vi "Group Analyser.vi"() -> ()   [LabVIEW 2016]
uses:
  Group Analyser state.ctl
  comm/comm.lvlib
  comm/impulse/impulse functions.lvlib
panel:
  in  "Fixed Time":bool
  in  "Fixed Time":bool
  in  "Active Plot":u16(ring) items=["BOTTOM PLOT", "TOP PLOT"]
  in  "Old Channels / Subject":T1(array[cluster])=[[{"Start"=0, "End"=1000000, "Offset"=0.0, "Deleted"=FALSE}]] {"Offset" format="%.2f"}
  in  "Channels / Subject":T1(array[cluster])=[[{"Start"=0, "End"=1000000, "Offset"=0.0, "Deleted"=FALSE}]] {"Offset" format="%.2f"}
  in  "Vertical Align to Zero":bool
  in  "Fixed Amplitude":bool
  out "Impulse Trace":cluster{dbl, dbl, dbl[][]}(graph)
  in  "Selected Files Text":string[](array[string])
  in  "Data Input":T2(array[cluster]) {"Data Channels" format="%.2f"}
  in  "Listbox":i32[](listbox)
  in  "Group Analyser":bool
  in  "Export Data":bool
  in  "Aligning Channel":u16(ring)=6 items=["Rx Position-in-Space", "Ry Position-in-Space", "Rz Position-in-Space", "Rx Velocity-in-Space", "Ry Velocity-in-Space", "Rz Velocity-in-Space", "Rl Velocity-in-Space", "Rr Velocity-in-Space", "Rx Acceleration-in-Space", "Ry Acceleration-in-Space", "Rz Acceleration-in-Space", "Rl Acceleration-in-Space", "Rr Acceleration-in-Space", "Chair Position", "Chair Velocity", " "]
  in  "Trigger Channel":u16(ring) items=["Rx Position-in-Space", "Ry Position-in-Space", "Rz Position-in-Space", "Rx Velocity-in-Space", "Ry Velocity-in-Space", "Rz Velocity-in-Space", "Rl Velocity-in-Space", "Rr Velocity-in-Space", "Rx Acceleration-in-Space", "Ry Acceleration-in-Space", "Rz Acceleration-in-Space", "Rl Acceleration-in-Space", "Rr Acceleration-in-Space", "Chair Position", "Chair Velocity", " "]
  in  "Plot Selection 2":T3(array[cluster])=[{"Color Box"=4652800, "Boolean"=TRUE, "List 2"=7, "Boolean 2"=FALSE}, {"Color Box"=16733696, "Boolean"=TRUE, "List 2"=15, "Boolean 2"=TRUE}, {"Color Box"=393436, "Boolean"=TRUE, "List 2"=23, "Boolean 2"=TRUE}] {"List 2" items=["Rx Position-in-Space", "Ry Position-in-Space", "Rz Position-in-Space", "Rx Velocity-in-Space", "Ry Velocity-in-Space", "Rz Velocity-in-Space", "Rl Velocity-in-Space", "Rr Velocity-in-Space", "Rx Acceleration-in-Space", "Ry Acceleration-in-Space", "Rz Acceleration-in-Space", "Rl Acceleration-in-Space", "Rr Acceleration-in-Space", "Chair Position", "Chair Velocity", " "]}
  in  "Select An  Other Trigger":bool
  in  "Group \nAnalyser":bool
  out "Processing":bool
  in  "View Impulse Parameters":bool
  in  "Filter Data":bool
  in  "View Filter Parameters":bool
  in  "Read Files":bool
  in  "Impulse Analyser":bool
  in  "Filter characteristics":T4={"Filter type"=enum."Lowpass", "Order"=50, "Higher pass freq"=40.0, "Lower pass freq"=40.0} {"Lower pass freq" format="%.2f"; "Higher pass freq" format="%.2f"}
  in  "Mean and STD":bool
  in  "Fixed Amplitude":bool
  in  "Cut After":bool
  in  "Cut Before":bool
  in  "Undo Last":bool
  in  "Delete Impulse":bool
  out "Impulse Trace":cluster{dbl, dbl, dbl[][]}(graph)
  in  "Vertical Align":bool
  in  "Horizontal Align":bool
  in  "Generate New Impulse Plot":bool
  in  "Select Files":bool
  in  "Plot Selection":T5(array[cluster])=[{"Color Box"=61223, "Boolean"=TRUE, "List 1"=5, "Boolean 2"=FALSE}, {"Color Box"=16722176, "Boolean"=TRUE, "List 1"=6, "Boolean 2"=FALSE}, {"Color Box"=6143, "Boolean"=TRUE, "List 1"=7, "Boolean 2"=FALSE}] {"List 1" items=["Rx Position-in-Space", "Ry Position-in-Space", "Rz Position-in-Space", "Rx Velocity-in-Space", "Ry Velocity-in-Space", "Rz Velocity-in-Space", "Rl Velocity-in-Space", "Rr Velocity-in-Space", "Rx Acceleration-in-Space", "Ry Acceleration-in-Space", "Rz Acceleration-in-Space", "Rl Acceleration-in-Space", "Rr Acceleration-in-Space", "Chair Position", "Chair Velocity", " "]}
  in  "Quit":bool
  in  "Stop":bool
  # "Copyright Americo A. Migliaccio (c) 2002 All Rights Reserved by Author"
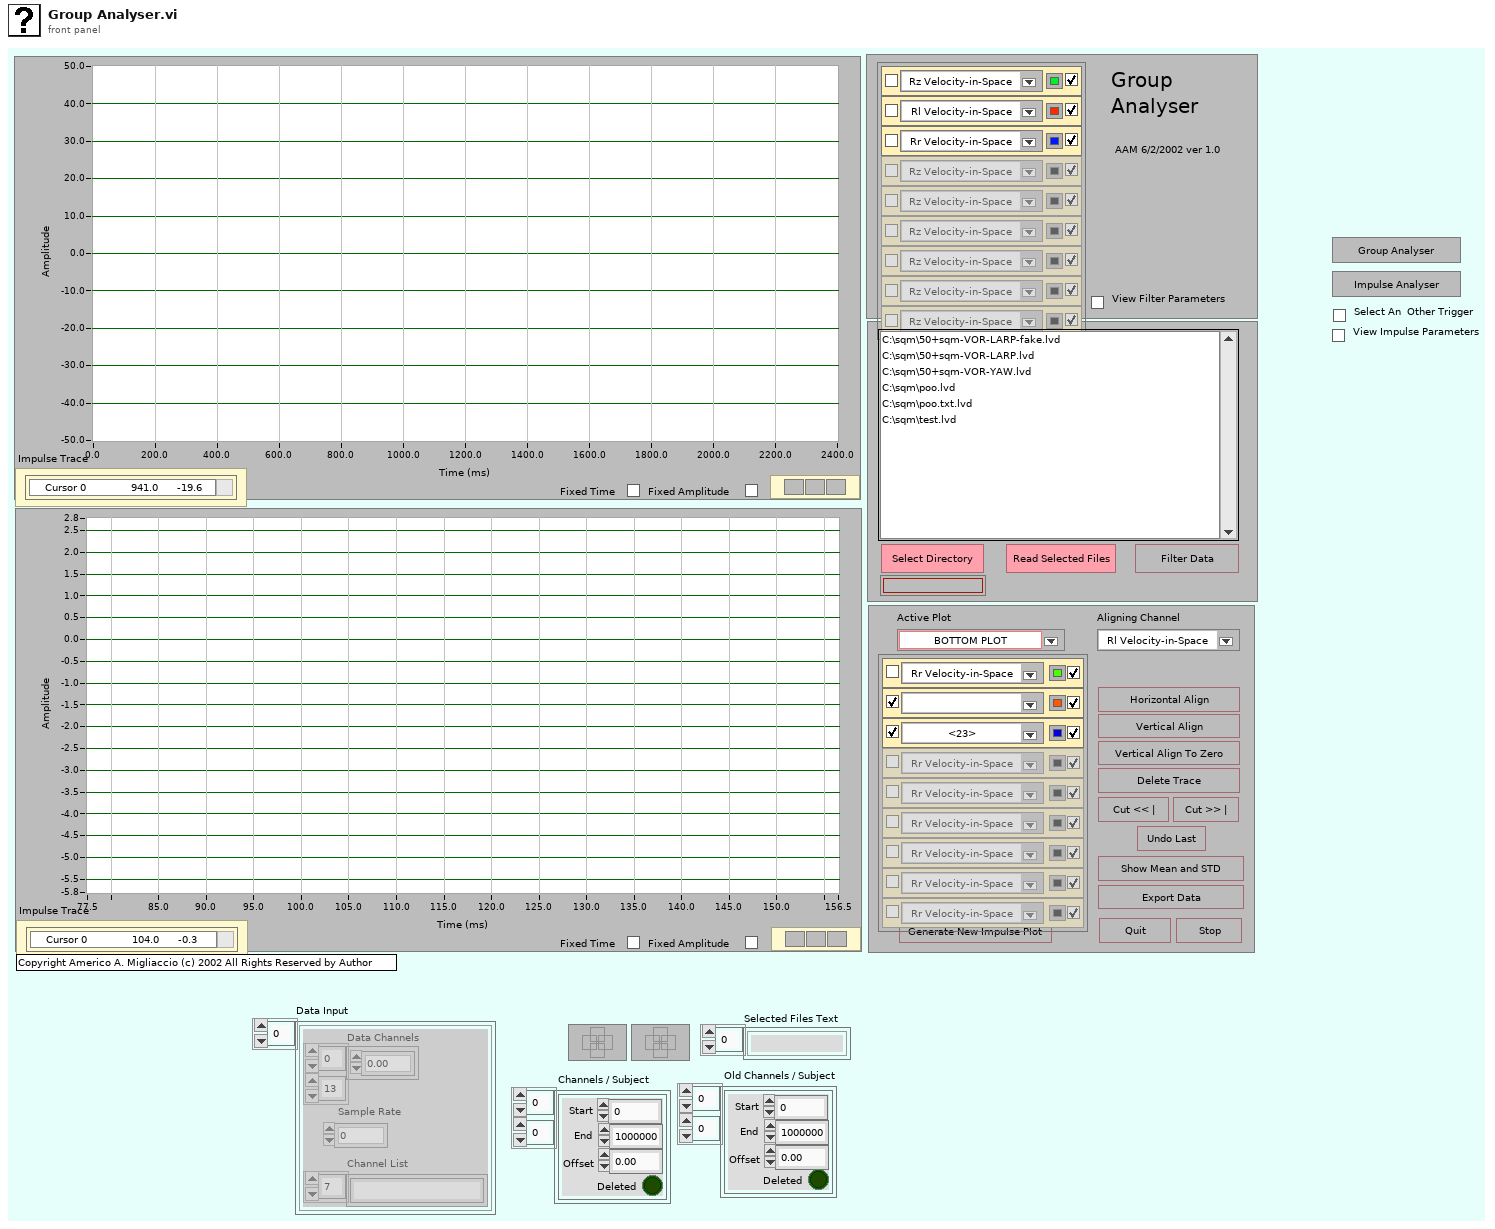
[diagram p1: front panel]
types:
  T1 = cluster{"Start":i32, "End":i32, "Offset":dbl, "Deleted":bool}[][]
  T2 = cluster{"Data Channels":dbl[][], "Sample Rate":i32, "Channel List":string[]}[]
  T3 = cluster{"Color Box":u32, "Boolean":bool, "List 2":u16, "Boolean 2":bool}[]
  T4 = cluster{"Filter type":enum32{"Lowpass", "Highpass", "Bandpass", "Bandstop"}, "Order":i32, "Higher pass freq":dbl, "Lower pass freq":dbl}
  T5 = cluster{"Color Box":u32, "Boolean":bool, "List 1":u16, "Boolean 2":bool}[]
  T6 = typedef "Group Analyser state.ctl" = enum16{"Panel Monitoring", "Read Files", "Select Files", "Generate New Impulse Plot", "Impulse Analyser", "Horizontal Align", "Vertical Align", "Vertical Align to Zero", "Delete Trace", "Cut Before", "Cut After", "Filter Data", "Undo Last", "Mean and STD", "Generate Report", "Export Data", "Initialize", "Stop", "Quit"}
  T7 = cluster{"Start":i32, "End":i32, "Offset":i32, "Deleted":bool}
  T8 = enum16{"open", "open or create", "create or replace", "create", "open (read only)"}
  T9 = cluster{"Data Input":cluster{"Data Channels":dbl[][], "Sample Rate":i32, "Channel List":string[]}[], "Selected Files Text":string[], " Channels / Subject":cluster{"Start":i32, "End":i32, "Offset":dbl, "Deleted":bool}[][], " Old Channels / Subject":cluster{"Start":i32, "End":i32, "Offset":dbl, "Deleted":bool}[][]}
  T10 = cluster{"Stop ":bool, "Quit":bool, "Read Files":bool, "Impulse Analyser":bool, "Select Files":bool, "View Filter Parameters":bool, "Filter Data":bool, "Generate New Impulse Plot":bool, "Vertical Align to Zero":bool, "Horizontal Align":bool, "Vertical Align":bool, "Delete Impulse":bool, "Undo Last":bool, "Cut Before":bool, "Cut After":bool, "Mean and STD":bool, "Select An  Other Trigger":bool, "Export Data":bool}
  T11 = enum32{"existing file", "new file", "new or existing file", "existing dir", "new dir", "new or existing dir", "existing file (use LLBs)", "new file (use LLBs)", "new or existing file (use LLBs)", "new or existing file or directory (use LLBs)"}
  T12 = cluster{"Data Channels":dbl[][], "Sample Rate":i32, "Channel List":string[]}
  T13 = cluster{"Start":i32, "End":i32, "Offset":i32, "Deleted":bool}[][]
  T14 = enum32{"Lowpass", "Highpass", "Bandpass", "Bandstop"}
  T15 = cluster{"Start":i32, "End":i32, "Offset":dbl, "Deleted":bool}
  T16 = cluster{"Color Box":u32, "Boolean":bool, "List 2":u16, "Boolean 2":bool}
  T17 = cluster{"Color Box":u32, "Boolean":bool, "List 1":u16, "Boolean 2":bool}
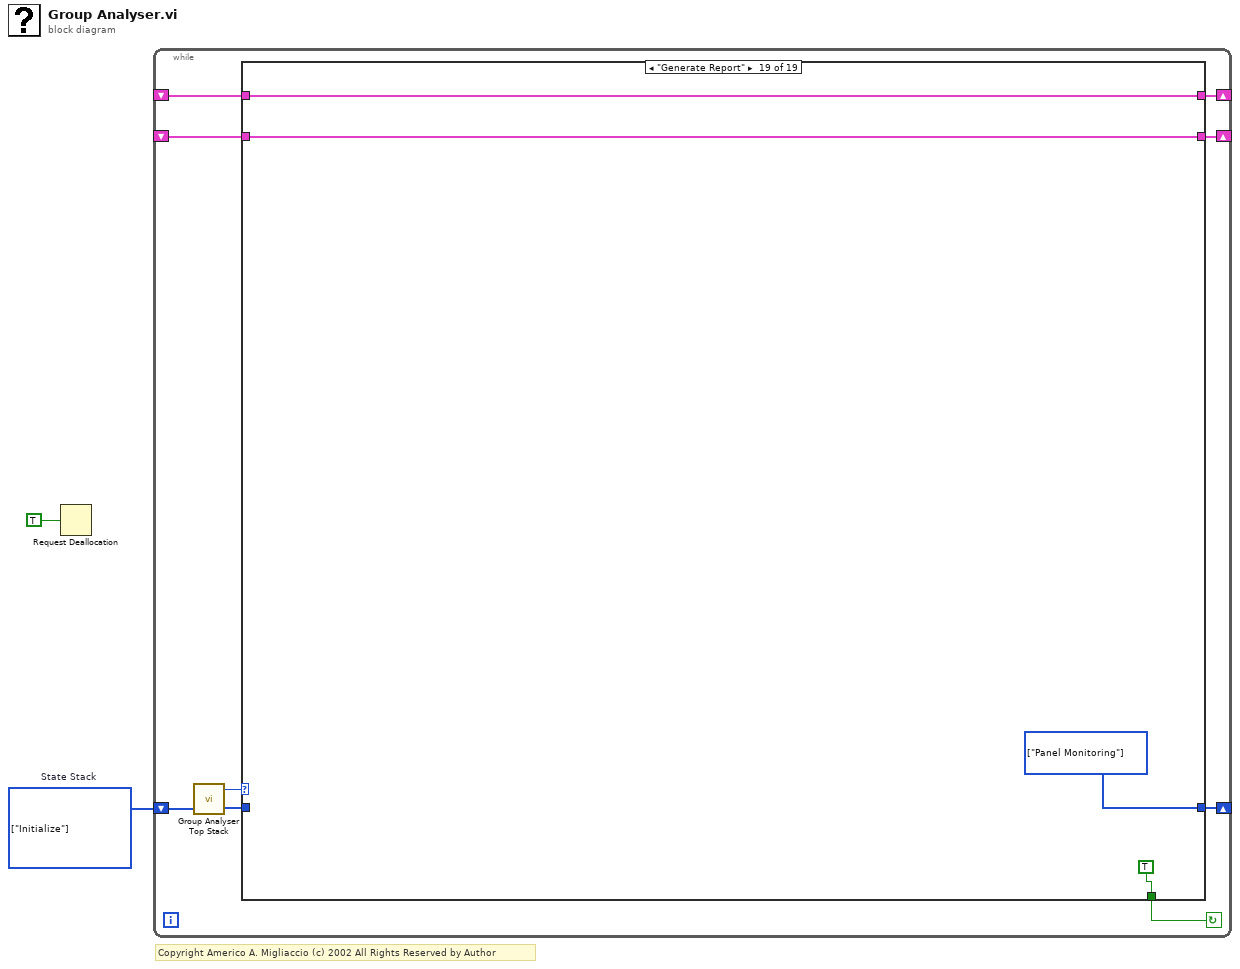
[diagram p0: block diagram]
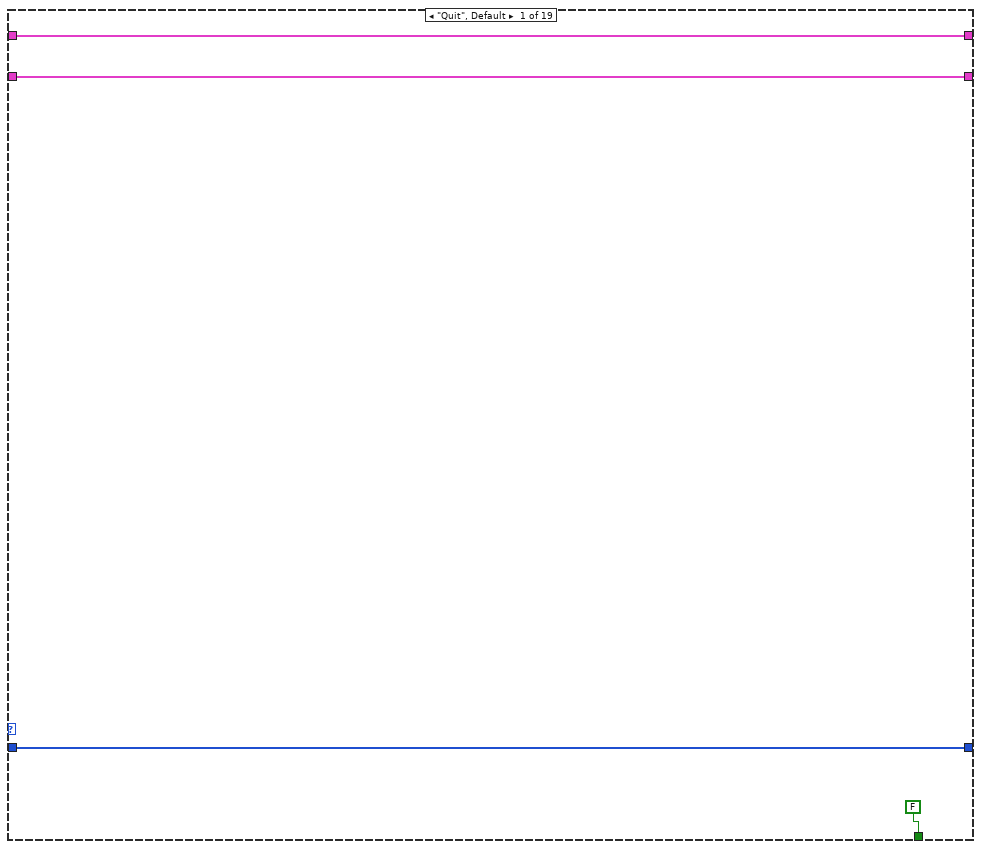
[diagram p2: hidden frame]
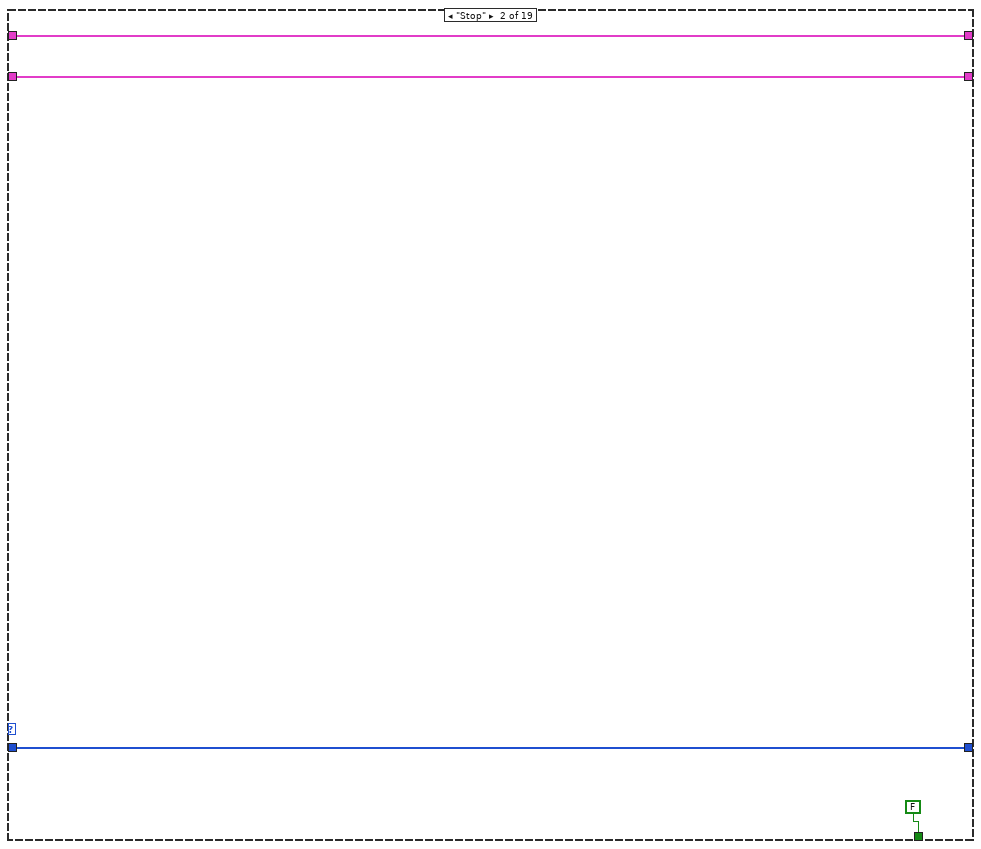
[diagram p3: hidden frame]
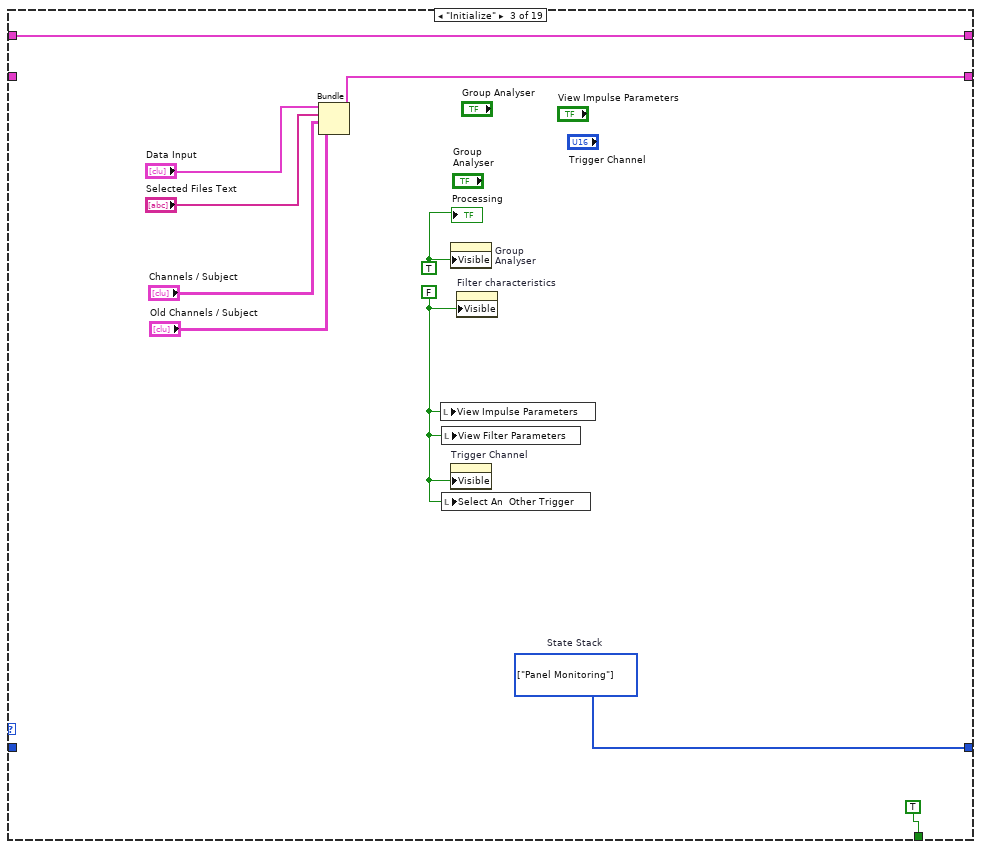
[diagram p4: hidden frame]
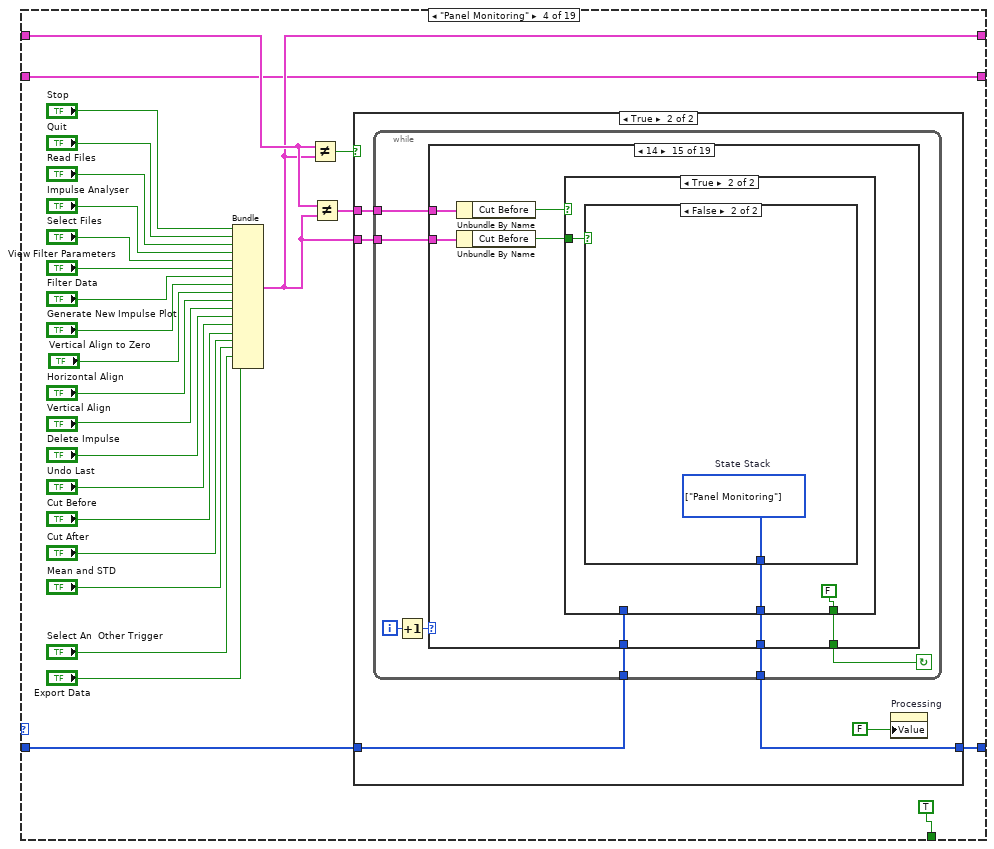
[diagram p5: hidden frame]
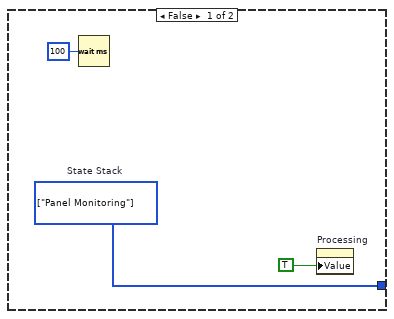
[diagram p6: hidden frame]
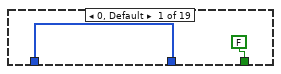
[diagram p7: hidden frame]
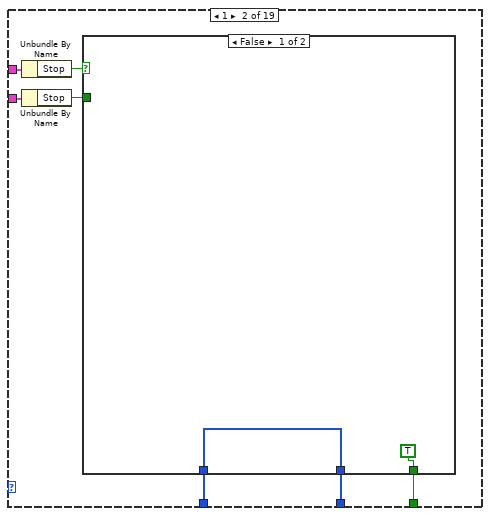
[diagram p8: hidden frame]
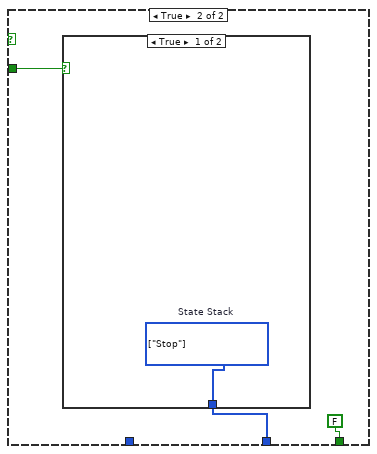
[diagram p9: hidden frame]
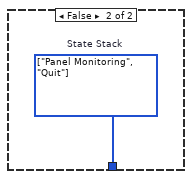
[diagram p10: hidden frame]
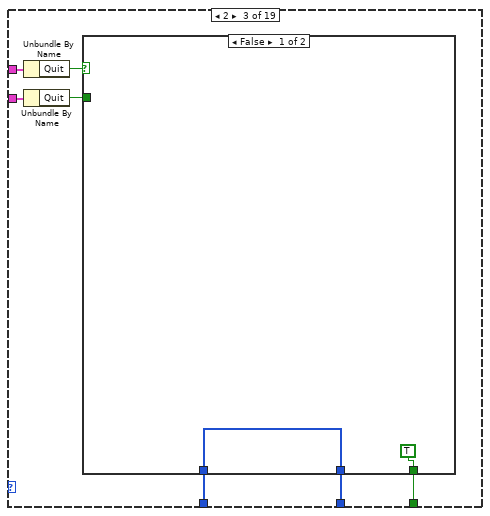
[diagram p11: hidden frame]
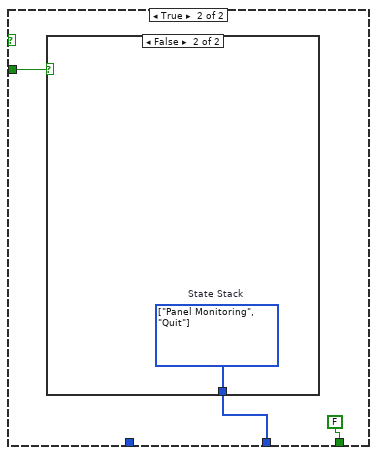
[diagram p12: hidden frame]
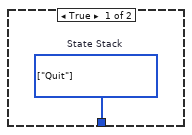
[diagram p13: hidden frame]
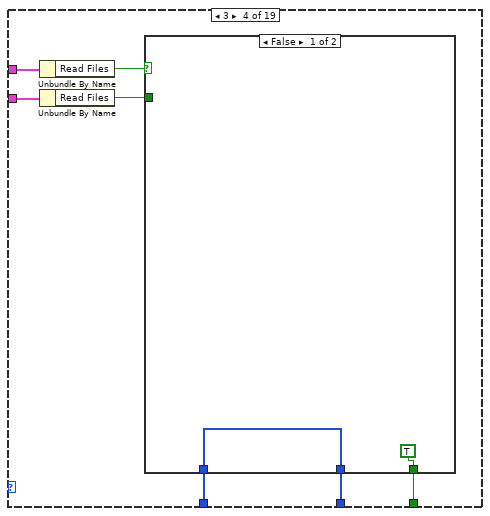
[diagram p14: hidden frame]
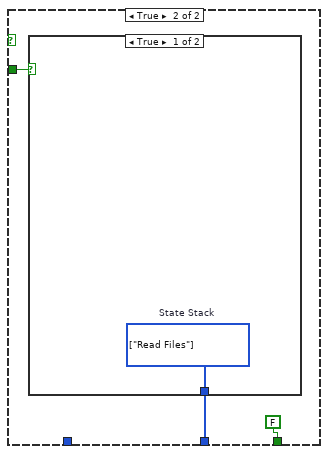
[diagram p15: hidden frame]
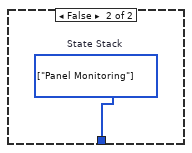
[diagram p16: hidden frame]
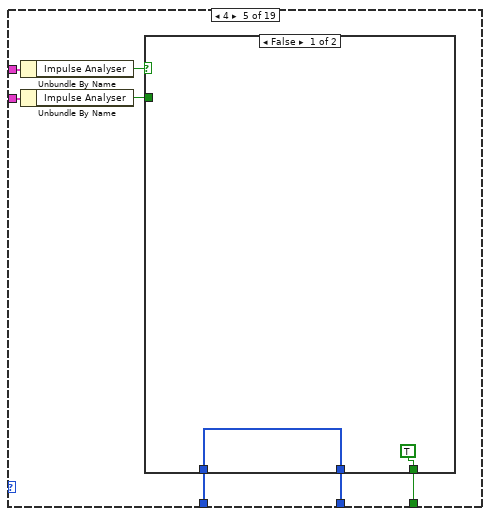
[diagram p17: hidden frame]
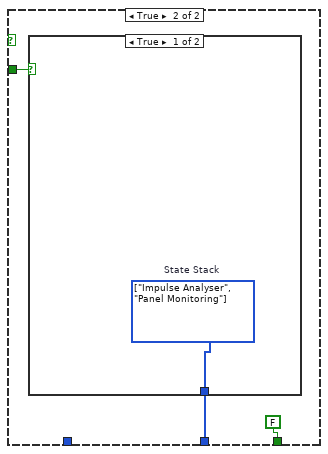
[diagram p18: hidden frame]
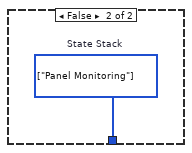
[diagram p19: hidden frame]
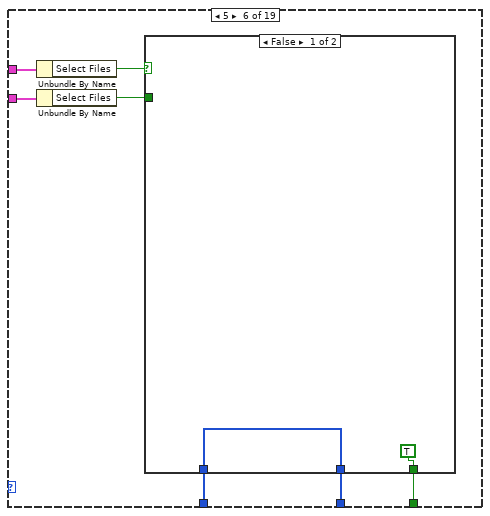
[diagram p20: hidden frame]
diagram:
  w2 = T6[] [enum."Initialize"] items=["Panel Monitoring", "Read Files", "Select Files", "Generate New Impulse Plot", "Impulse Analyser", "Horizontal Align", "Vertical Align", "Vertical Align to Zero", "Delete Trace", "Cut Before", "Cut After", "Filter Data", "Undo Last", "Mean and STD", "Generate Report", "Export Data", "Initialize", "Stop", "Quit"]  # State Stack
  # "Copyright Americo A. Migliaccio (c) 2002 All Rights Reserved by Author"
  n1 = Request Deallocation(TRUE ("flag")) -> ()
  n2 = while {
    shift-left: _ -> [w4]
    shift-right: [w5] -> _
    shift-left: _ -> [w7]
    shift-right: [w8] -> _
    shift-left: w2 -> [w11]
    shift-right: [w9] -> _
    stop <- w6 continue-if-true
    n3 = call "Group Analyser Top Stack.vi"("State Stack (in)"=w11) -> ("State Stack (out)"=w10:T6[], "State"=w3:T6)  [unwired: 1 in]
    n4 = case shown="\"Generate Report\"" w3 {
      tunnel: w10 -> [w15 w19 _ w50 _ _ w375 _ w490 w507 w522 w538 w570 w592 w610 _ w695 _ _]
      tunnel: [w15 w19 w28 w49 w335 w357 w375 w403 w490 w507 w522 w538 w570 w592 w610 w636 w695 w742 w753] -> w9
      tunnel: [w13 w17 w27 w46 w336 w358 w382 w404 w491 w508 w523 w540 w571 w595 w611 w637 w696 w743 w754] -> w8
      tunnel: w7 -> [w13 w17 w27 w52 w336 w358 w382 w404 w491 w508 w523 w540 w571 w595 w611 w637 w696 w743 w754]
      tunnel: [FALSE FALSE TRUE TRUE TRUE TRUE TRUE TRUE TRUE TRUE TRUE TRUE TRUE TRUE TRUE TRUE TRUE TRUE TRUE] -> w6
      tunnel: [w12 w16 w24 w33 w326 w350 w372 w398 w488 w503 w519 w539 w562 w593 w608 w631 w694 w741 w752] -> w5
      tunnel: w4 -> [w12 w16 _ w33 w328 w356 w373 w398 w489 w504 w520 w537 w563 w594 w609 w631 w694 w741 w752]
      frame "Quit", Default {
      }
      frame "Stop" {
      }
      frame "Initialize" {
        w28 = T6[] [enum."Panel Monitoring"] items=["Panel Monitoring", "Read Files", "Select Files", "Generate New Impulse Plot", "Impulse Analyser", "Horizontal Align", "Vertical Align", "Vertical Align to Zero", "Delete Trace", "Cut Before", "Cut After", "Filter Data", "Undo Last", "Mean and STD", "Generate Report", "Export Data", "Initialize", "Stop", "Quit"]  # State Stack
        w26 = TRUE ("Visible")
        w25 = FALSE
        n5 = Bundle("Data Input"="Data Input", "Selected Files Text"="Selected Files Text", "Channels / Subject"="Channels / Subject", "Old Channels / Subject"="Old Channels / Subject") -> (w24:T9)  [unwired: 1 in]
        n6 = local write "View Impulse Parameters"(w25) -> ()
        n7 = local write "View Filter Parameters"(w25) -> ()
        n8 = local write "Select An  Other Trigger"(w25) -> ()
        n9 = property on="Group \nAnalyser" class="Bool"("Visible"=w26) -> ()  [unwired: 2 in, 2 out]
        n10 = property on="Trigger Channel" class="Ring (strict)"("Visible"=w25) -> ()  [unwired: 2 in, 2 out]
        n11 = property on="Filter characteristics" class="Clust (strict)"("Visible"=w25) -> ()  [unwired: 2 in, 2 out]
        "Processing" <- w26
      }
      frame "Panel Monitoring" {
        n12 = Bundle("Stop"="Stop", "Quit"="Quit", "Read Files"="Read Files", "Impulse Analyser"="Impulse Analyser", "Select Files"="Select Files", "View Filter Parameters"="View Filter Parameters", "Filter Data"="Filter Data", "Generate New Impulse Plot"="Generate New Impulse Plot", "Vertical Align to Zero"="Vertical Align to Zero", "Horizontal Align"="Horizontal Align", "Vertical Align"="Vertical Align", "Delete Impulse"="Delete Impulse", "Undo Last"="Undo Last", "Cut Before"="Cut Before", "Cut After"="Cut After", "Mean and STD"="Mean and STD", "Select An  Other Trigger"="Select An  Other Trigger", "Export Data"="Export Data") -> (w46:T10)  [unwired: 1 in]
        n13 = Not Equal?(x=w52, y=w46) -> (x != y?=w53:bool)
        n14 = Not Equal?(x=w52, y=w46) -> (x != y?=w51:T10)
        n15 = case shown="True" w53 {
          tunnel: w51 -> [_ w63]
          tunnel: w50 -> [_ w61]
          tunnel: [w58 w62] -> w49
          tunnel: w46 -> [_ w60]
          frame False {
            w58 = T6[] [enum."Panel Monitoring"] items=["Panel Monitoring", "Read Files", "Select Files", "Generate New Impulse Plot", "Impulse Analyser", "Horizontal Align", "Vertical Align", "Vertical Align to Zero", "Delete Trace", "Cut Before", "Cut After", "Filter Data", "Undo Last", "Mean and STD", "Generate Report", "Export Data", "Initialize", "Stop", "Quit"]  # State Stack
            n16 = Wait (ms)(milliseconds to wait=u32 100) -> ()  [unwired: 1 out]
            n17 = property on="Processing" class="Bool (strict)"("Value"=TRUE) -> ()  [unwired: 2 in, 2 out]
          }
          frame True {
            n18 = while {
              tunnel: w60 -> [w64]
              tunnel: w61 -> [w67]
              tunnel: [w68] -> w62
              tunnel: w63 -> [w70]
              i -> [w69]
              stop <- w66 continue-if-true
              n19 = Increment(x=w69) -> (x+1=w65:i32)
              n20 = case shown="14" w65 {
                tunnel: w70 -> [_ w79 w93 w107 w121 w135 w149 w162 w176 w190 w204 w218 w232 w246 w260 w274 w288 w303 w317]
                tunnel: [w72 w77 w91 w105 w119 w133 w147 w160 w174 w188 w202 w216 w230 w244 w258 w272 w286 w301 w315] -> w68
                tunnel: w67 -> [w72 w76 w90 w104 w118 w132 w146 w159 w173 w187 w201 w215 w229 w243 w257 w271 w285 w300 w314]
                tunnel: [FALSE w75 w89 w103 w117 w131 w145 w158 w172 w186 w200 w214 w228 w242 w256 w270 w284 w299 w313] -> w66
                tunnel: w64 -> [_ w74 w88 w102 w116 w130 w144 w157 w171 w185 w199 w213 w227 w241 w255 w269 w283 w298 w312]
                frame 0, Default {
                }
                frame 1 {
                  n21 = Unbundle By Name(w79) -> ("Stop"=w78:bool)
                  n22 = Unbundle By Name(w74) -> ("Stop"=w73:bool)
                  n23 = case shown="False" w78 {
                    tunnel: [w81 w84] -> w77
                    tunnel: w76 -> [w81 _]
                    tunnel: [TRUE FALSE] -> w75
                    tunnel: w73 -> [_ w82]
                    frame False {
                    }
                    frame True {
                      n24 = case shown="True" w82 {
                        tunnel: [w85 w86] -> w84
                        frame True {
                          w85 = T6[] [enum."Stop"] items=["Panel Monitoring", "Read Files", "Select Files", "Generate New Impulse Plot", "Impulse Analyser", "Horizontal Align", "Vertical Align", "Vertical Align to Zero", "Delete Trace", "Cut Before", "Cut After", "Filter Data", "Undo Last", "Mean and STD", "Generate Report", "Export Data", "Initialize", "Stop", "Quit"]  # State Stack
                        }
                        frame False {
                          w86 = T6[] [enum."Panel Monitoring", enum."Quit"] items=["Panel Monitoring", "Read Files", "Select Files", "Generate New Impulse Plot", "Impulse Analyser", "Horizontal Align", "Vertical Align", "Vertical Align to Zero", "Delete Trace", "Cut Before", "Cut After", "Filter Data", "Undo Last", "Mean and STD", "Generate Report", "Export Data", "Initialize", "Stop", "Quit"]  # State Stack
                        }
                      }
                    }
                  }
                }
                frame 2 {
                  n25 = Unbundle By Name(w93) -> ("Quit"=w92:bool)
                  n26 = Unbundle By Name(w88) -> ("Quit"=w87:bool)
                  n27 = case shown="False" w92 {
                    tunnel: [w95 w98] -> w91
                    tunnel: w90 -> [w95 _]
                    tunnel: [TRUE FALSE] -> w89
                    tunnel: w87 -> [_ w96]
                    frame False {
                    }
                    frame True {
                      n28 = case shown="False" w96 {
                        tunnel: [w99 w100] -> w98
                        frame True {
                          w99 = T6[] [enum."Quit"] items=["Panel Monitoring", "Read Files", "Select Files", "Generate New Impulse Plot", "Impulse Analyser", "Horizontal Align", "Vertical Align", "Vertical Align to Zero", "Delete Trace", "Cut Before", "Cut After", "Filter Data", "Undo Last", "Mean and STD", "Generate Report", "Export Data", "Initialize", "Stop", "Quit"]  # State Stack
                        }
                        frame False {
                          w100 = T6[] [enum."Panel Monitoring", enum."Quit"] items=["Panel Monitoring", "Read Files", "Select Files", "Generate New Impulse Plot", "Impulse Analyser", "Horizontal Align", "Vertical Align", "Vertical Align to Zero", "Delete Trace", "Cut Before", "Cut After", "Filter Data", "Undo Last", "Mean and STD", "Generate Report", "Export Data", "Initialize", "Stop", "Quit"]  # State Stack
                        }
                      }
                    }
                  }
                }
                frame 3 {
                  n29 = Unbundle By Name(w107) -> ("Read Files"=w106:bool)
                  n30 = Unbundle By Name(w102) -> ("Read Files"=w101:bool)
                  n31 = case shown="False" w106 {
                    tunnel: [w109 w112] -> w105
                    tunnel: w104 -> [w109 _]
                    tunnel: [TRUE FALSE] -> w103
                    tunnel: w101 -> [_ w110]
                    frame False {
                    }
                    frame True {
                      n32 = case shown="True" w110 {
                        tunnel: [w113 w114] -> w112
                        frame True {
                          w113 = T6[] [enum."Read Files"] items=["Panel Monitoring", "Read Files", "Select Files", "Generate New Impulse Plot", "Impulse Analyser", "Horizontal Align", "Vertical Align", "Vertical Align to Zero", "Delete Trace", "Cut Before", "Cut After", "Filter Data", "Undo Last", "Mean and STD", "Generate Report", "Export Data", "Initialize", "Stop", "Quit"]  # State Stack
                        }
                        frame False {
                          w114 = T6[] [enum."Panel Monitoring"] items=["Panel Monitoring", "Read Files", "Select Files", "Generate New Impulse Plot", "Impulse Analyser", "Horizontal Align", "Vertical Align", "Vertical Align to Zero", "Delete Trace", "Cut Before", "Cut After", "Filter Data", "Undo Last", "Mean and STD", "Generate Report", "Export Data", "Initialize", "Stop", "Quit"]  # State Stack
                        }
                      }
                    }
                  }
                }
                frame 4 {
                  n33 = Unbundle By Name(w121) -> ("Impulse Analyser"=w120:bool)
                  n34 = Unbundle By Name(w116) -> ("Impulse Analyser"=w115:bool)
                  n35 = case shown="False" w120 {
                    tunnel: [w123 w126] -> w119
                    tunnel: w118 -> [w123 _]
                    tunnel: [TRUE FALSE] -> w117
                    tunnel: w115 -> [_ w124]
                    frame False {
                    }
                    frame True {
                      n36 = case shown="True" w124 {
                        tunnel: [w127 w128] -> w126
                        frame True {
                          w127 = T6[] [enum."Impulse Analyser", enum."Panel Monitoring"] items=["Panel Monitoring", "Read Files", "Select Files", "Generate New Impulse Plot", "Impulse Analyser", "Horizontal Align", "Vertical Align", "Vertical Align to Zero", "Delete Trace", "Cut Before", "Cut After", "Filter Data", "Undo Last", "Mean and STD", "Generate Report", "Export Data", "Initialize", "Stop", "Quit"]  # State Stack
                        }
                        frame False {
                          w128 = T6[] [enum."Panel Monitoring"] items=["Panel Monitoring", "Read Files", "Select Files", "Generate New Impulse Plot", "Impulse Analyser", "Horizontal Align", "Vertical Align", "Vertical Align to Zero", "Delete Trace", "Cut Before", "Cut After", "Filter Data", "Undo Last", "Mean and STD", "Generate Report", "Export Data", "Initialize", "Stop", "Quit"]  # State Stack
                        }
                      }
                    }
                  }
                }
                frame 5 {
                  n37 = Unbundle By Name(w135) -> ("Select Files"=w134:bool)
                  n38 = Unbundle By Name(w130) -> ("Select Files"=w129:bool)
                  n39 = case shown="False" w134 {
                    tunnel: [w137 w140] -> w133
                    tunnel: w132 -> [w137 _]
                    tunnel: [TRUE FALSE] -> w131
                    tunnel: w129 -> [_ w138]
                    frame False {
                    }
                    frame True {
                      n40 = case shown="True" w138 {
                        tunnel: [w141 w142] -> w140
                        frame True {
                          w141 = T6[] [enum."Select Files"] items=["Panel Monitoring", "Read Files", "Select Files", "Generate New Impulse Plot", "Impulse Analyser", "Horizontal Align", "Vertical Align", "Vertical Align to Zero", "Delete Trace", "Cut Before", "Cut After", "Filter Data", "Undo Last", "Mean and STD", "Generate Report", "Export Data", "Initialize", "Stop", "Quit"]  # State Stack
                        }
                        frame False {
                          w142 = T6[] [enum."Panel Monitoring"] items=["Panel Monitoring", "Read Files", "Select Files", "Generate New Impulse Plot", "Impulse Analyser", "Horizontal Align", "Vertical Align", "Vertical Align to Zero", "Delete Trace", "Cut Before", "Cut After", "Filter Data", "Undo Last", "Mean and STD", "Generate Report", "Export Data", "Initialize", "Stop", "Quit"]  # State Stack
                        }
                      }
                    }
                  }
                }
                frame 6 {
                  n41 = Unbundle By Name(w149) -> ("View Filter Parameters"=w148:bool)
                  n42 = Unbundle By Name(w144) -> ("View Filter Parameters"=w143:bool)
                  n43 = case shown="True" w148 {
                    tunnel: [w151 w154] -> w147
                    tunnel: w146 -> [w151 _]
                    tunnel: [TRUE FALSE] -> w145
                    tunnel: w143 -> [_ w152]
                    frame False {
                    }
                    frame True {
                      w154 = T6[] [enum."Panel Monitoring"] items=["Panel Monitoring", "Read Files", "Select Files", "Generate New Impulse Plot", "Impulse Analyser", "Horizontal Align", "Vertical Align", "Vertical Align to Zero", "Delete Trace", "Cut Before", "Cut After", "Filter Data", "Undo Last", "Mean and STD", "Generate Report", "Export Data", "Initialize", "Stop", "Quit"]  # State Stack
                      n44 = Not(x=w152) -> (.not. x?=w153:bool)
                      n45 = property on="Filter characteristics" class="Clust (strict)"("Visible"=w152) -> ()  [unwired: 2 in, 2 out]
                      n46 = property on="Group \nAnalyser" class="Bool"("Visible"=w153) -> ()  [unwired: 2 in, 2 out]
                    }
                  }
                }
                frame 7 {
                  n47 = Unbundle By Name(w162) -> ("Filter Data"=w161:bool)
                  n48 = Unbundle By Name(w157) -> ("Filter Data"=w156:bool)
                  n49 = case shown="False" w161 {
                    tunnel: [w164 w167] -> w160
                    tunnel: w159 -> [w164 _]
                    tunnel: [TRUE FALSE] -> w158
                    tunnel: w156 -> [_ w165]
                    frame False {
                    }
                    frame True {
                      n50 = case shown="True" w165 {
                        tunnel: [w168 w169] -> w167
                        frame True {
                          w168 = T6[] [enum."Filter Data", enum."Select Files"] items=["Panel Monitoring", "Read Files", "Select Files", "Generate New Impulse Plot", "Impulse Analyser", "Horizontal Align", "Vertical Align", "Vertical Align to Zero", "Delete Trace", "Cut Before", "Cut After", "Filter Data", "Undo Last", "Mean and STD", "Generate Report", "Export Data", "Initialize", "Stop", "Quit"]  # State Stack
                        }
                        frame False {
                          w169 = T6[] [enum."Panel Monitoring"] items=["Panel Monitoring", "Read Files", "Select Files", "Generate New Impulse Plot", "Impulse Analyser", "Horizontal Align", "Vertical Align", "Vertical Align to Zero", "Delete Trace", "Cut Before", "Cut After", "Filter Data", "Undo Last", "Mean and STD", "Generate Report", "Export Data", "Initialize", "Stop", "Quit"]  # State Stack
                        }
                      }
                    }
                  }
                }
                frame 8 {
                  n51 = Unbundle By Name(w176) -> ("Generate New Impulse Plot"=w175:bool)
                  n52 = Unbundle By Name(w171) -> ("Generate New Impulse Plot"=w170:bool)
                  n53 = case shown="True" w175 {
                    tunnel: [w178 w181] -> w174
                    tunnel: w173 -> [w178 _]
                    tunnel: [TRUE FALSE] -> w172
                    tunnel: w170 -> [_ w179]
                    frame False {
                    }
                    frame True {
                      n54 = case shown="False" w179 {
                        tunnel: [w182 w183] -> w181
                        frame True {
                          w182 = T6[] [enum."Generate New Impulse Plot"] items=["Panel Monitoring", "Read Files", "Select Files", "Generate New Impulse Plot", "Impulse Analyser", "Horizontal Align", "Vertical Align", "Vertical Align to Zero", "Delete Trace", "Cut Before", "Cut After", "Filter Data", "Undo Last", "Mean and STD", "Generate Report", "Export Data", "Initialize", "Stop", "Quit"]  # State Stack
                        }
                        frame False {
                          w183 = T6[] [enum."Panel Monitoring"] items=["Panel Monitoring", "Read Files", "Select Files", "Generate New Impulse Plot", "Impulse Analyser", "Horizontal Align", "Vertical Align", "Vertical Align to Zero", "Delete Trace", "Cut Before", "Cut After", "Filter Data", "Undo Last", "Mean and STD", "Generate Report", "Export Data", "Initialize", "Stop", "Quit"]  # State Stack
                        }
                      }
                    }
                  }
                }
                frame 9 {
                  n55 = Unbundle By Name(w190) -> ("Vertical Align to Zero"=w189:bool)
                  n56 = Unbundle By Name(w185) -> ("Vertical Align to Zero"=w184:bool)
                  n57 = case shown="True" w189 {
                    tunnel: [w192 w194] -> w188
                    tunnel: w187 -> [w192 _]
                    tunnel: [TRUE FALSE] -> w186
                    tunnel: w184 -> [_ w193]
                    frame False {
                    }
                    frame True {
                      n58 = case shown="True" w193 {
                        tunnel: [w196 w197] -> w194
                        frame True {
                          w196 = T6[] [enum."Vertical Align to Zero", enum."Generate New Impulse Plot"] items=["Panel Monitoring", "Read Files", "Select Files", "Generate New Impulse Plot", "Impulse Analyser", "Horizontal Align", "Vertical Align", "Vertical Align to Zero", "Delete Trace", "Cut Before", "Cut After", "Filter Data", "Undo Last", "Mean and STD", "Generate Report", "Export Data", "Initialize", "Stop", "Quit"]  # State Stack
                        }
                        frame False {
                          w197 = T6[] [enum."Panel Monitoring"] items=["Panel Monitoring", "Read Files", "Select Files", "Generate New Impulse Plot", "Impulse Analyser", "Horizontal Align", "Vertical Align", "Vertical Align to Zero", "Delete Trace", "Cut Before", "Cut After", "Filter Data", "Undo Last", "Mean and STD", "Generate Report", "Export Data", "Initialize", "Stop", "Quit"]  # State Stack
                        }
                      }
                    }
                  }
                }
                frame 10 {
                  n59 = Unbundle By Name(w204) -> ("Horizontal Align"=w203:bool)
                  n60 = Unbundle By Name(w199) -> ("Horizontal Align"=w198:bool)
                  n61 = case shown="True" w203 {
                    tunnel: [w206 w209] -> w202
                    tunnel: w201 -> [w206 _]
                    tunnel: [TRUE FALSE] -> w200
                    tunnel: w198 -> [_ w207]
                    frame False {
                    }
                    frame True {
                      n62 = case shown="True" w207 {
                        tunnel: [w210 w211] -> w209
                        frame True {
                          w210 = T6[] [enum."Horizontal Align", enum."Generate New Impulse Plot"] items=["Panel Monitoring", "Read Files", "Select Files", "Generate New Impulse Plot", "Impulse Analyser", "Horizontal Align", "Vertical Align", "Vertical Align to Zero", "Delete Trace", "Cut Before", "Cut After", "Filter Data", "Undo Last", "Mean and STD", "Generate Report", "Export Data", "Initialize", "Stop", "Quit"]  # State Stack
                        }
                        frame False {
                          w211 = T6[] [enum."Panel Monitoring"] items=["Panel Monitoring", "Read Files", "Select Files", "Generate New Impulse Plot", "Impulse Analyser", "Horizontal Align", "Vertical Align", "Vertical Align to Zero", "Delete Trace", "Cut Before", "Cut After", "Filter Data", "Undo Last", "Mean and STD", "Generate Report", "Export Data", "Initialize", "Stop", "Quit"]  # State Stack
                        }
                      }
                    }
                  }
                }
                frame 11 {
                  n63 = Unbundle By Name(w218) -> ("Vertical Align"=w217:bool)
                  n64 = Unbundle By Name(w213) -> ("Vertical Align"=w212:bool)
                  n65 = case shown="True" w217 {
                    tunnel: [w220 w223] -> w216
                    tunnel: w215 -> [w220 _]
                    tunnel: [TRUE FALSE] -> w214
                    tunnel: w212 -> [_ w221]
                    frame False {
                    }
                    frame True {
                      n66 = case shown="True" w221 {
                        tunnel: [w224 w225] -> w223
                        frame True {
                          w224 = T6[] [enum."Vertical Align", enum."Generate New Impulse Plot"] items=["Panel Monitoring", "Read Files", "Select Files", "Generate New Impulse Plot", "Impulse Analyser", "Horizontal Align", "Vertical Align", "Vertical Align to Zero", "Delete Trace", "Cut Before", "Cut After", "Filter Data", "Undo Last", "Mean and STD", "Generate Report", "Export Data", "Initialize", "Stop", "Quit"]  # State Stack
                        }
                        frame False {
                          w225 = T6[] [enum."Panel Monitoring", enum."Quit"] items=["Panel Monitoring", "Read Files", "Select Files", "Generate New Impulse Plot", "Impulse Analyser", "Horizontal Align", "Vertical Align", "Vertical Align to Zero", "Delete Trace", "Cut Before", "Cut After", "Filter Data", "Undo Last", "Mean and STD", "Generate Report", "Export Data", "Initialize", "Stop", "Quit"]  # State Stack
                        }
                      }
                    }
                  }
                }
                frame 12 {
                  n67 = Unbundle By Name(w232) -> ("Delete Impulse"=w231:bool)
                  n68 = Unbundle By Name(w227) -> ("Delete Impulse"=w226:bool)
                  n69 = case shown="True" w231 {
                    tunnel: [w234 w237] -> w230
                    tunnel: w229 -> [w234 _]
                    tunnel: [TRUE FALSE] -> w228
                    tunnel: w226 -> [_ w235]
                    frame False {
                    }
                    frame True {
                      n70 = case shown="False" w235 {
                        tunnel: [w238 w239] -> w237
                        frame True {
                          w238 = T6[] [enum."Delete Trace", enum."Generate New Impulse Plot"] items=["Panel Monitoring", "Read Files", "Select Files", "Generate New Impulse Plot", "Impulse Analyser", "Horizontal Align", "Vertical Align", "Vertical Align to Zero", "Delete Trace", "Cut Before", "Cut After", "Filter Data", "Undo Last", "Mean and STD", "Generate Report", "Export Data", "Initialize", "Stop", "Quit"]  # State Stack
                        }
                        frame False {
                          w239 = T6[] [enum."Panel Monitoring"] items=["Panel Monitoring", "Read Files", "Select Files", "Generate New Impulse Plot", "Impulse Analyser", "Horizontal Align", "Vertical Align", "Vertical Align to Zero", "Delete Trace", "Cut Before", "Cut After", "Filter Data", "Undo Last", "Mean and STD", "Generate Report", "Export Data", "Initialize", "Stop", "Quit"]  # State Stack
                        }
                      }
                    }
                  }
                }
                frame 13 {
                  n71 = Unbundle By Name(w246) -> ("Undo Last"=w245:bool)
                  n72 = Unbundle By Name(w241) -> ("Undo Last"=w240:bool)
                  n73 = case shown="True" w245 {
                    tunnel: [w248 w251] -> w244
                    tunnel: w243 -> [w248 _]
                    tunnel: [TRUE FALSE] -> w242
                    tunnel: w240 -> [_ w249]
                    frame False {
                    }
                    frame True {
                      n74 = case shown="True" w249 {
                        tunnel: [w252 w253] -> w251
                        frame True {
                          w252 = T6[] [enum."Undo Last", enum."Generate New Impulse Plot"] items=["Panel Monitoring", "Read Files", "Select Files", "Generate New Impulse Plot", "Impulse Analyser", "Horizontal Align", "Vertical Align", "Vertical Align to Zero", "Delete Trace", "Cut Before", "Cut After", "Filter Data", "Undo Last", "Mean and STD", "Generate Report", "Export Data", "Initialize", "Stop", "Quit"]  # State Stack
                        }
                        frame False {
                          w253 = T6[] [enum."Panel Monitoring"] items=["Panel Monitoring", "Read Files", "Select Files", "Generate New Impulse Plot", "Impulse Analyser", "Horizontal Align", "Vertical Align", "Vertical Align to Zero", "Delete Trace", "Cut Before", "Cut After", "Filter Data", "Undo Last", "Mean and STD", "Generate Report", "Export Data", "Initialize", "Stop", "Quit"]  # State Stack
                        }
                      }
                    }
                  }
                }
                frame 14 {
                  n75 = Unbundle By Name(w260) -> ("Cut Before"=w259:bool)
                  n76 = Unbundle By Name(w255) -> ("Cut Before"=w254:bool)
                  n77 = case shown="True" w259 {
                    tunnel: [w262 w265] -> w258
                    tunnel: w257 -> [w262 _]
                    tunnel: [TRUE FALSE] -> w256
                    tunnel: w254 -> [_ w263]
                    frame False {
                    }
                    frame True {
                      n78 = case shown="False" w263 {
                        tunnel: [w266 w267] -> w265
                        frame True {
                          w266 = T6[] [enum."Cut Before", enum."Generate New Impulse Plot"] items=["Panel Monitoring", "Read Files", "Select Files", "Generate New Impulse Plot", "Impulse Analyser", "Horizontal Align", "Vertical Align", "Vertical Align to Zero", "Delete Trace", "Cut Before", "Cut After", "Filter Data", "Undo Last", "Mean and STD", "Generate Report", "Export Data", "Initialize", "Stop", "Quit"]  # State Stack
                        }
                        frame False {
                          w267 = T6[] [enum."Panel Monitoring"] items=["Panel Monitoring", "Read Files", "Select Files", "Generate New Impulse Plot", "Impulse Analyser", "Horizontal Align", "Vertical Align", "Vertical Align to Zero", "Delete Trace", "Cut Before", "Cut After", "Filter Data", "Undo Last", "Mean and STD", "Generate Report", "Export Data", "Initialize", "Stop", "Quit"]  # State Stack
                        }
                      }
                    }
                  }
                }
                frame 15 {
                  n79 = Unbundle By Name(w274) -> ("Cut After"=w273:bool)
                  n80 = Unbundle By Name(w269) -> ("Cut After"=w268:bool)
                  n81 = case shown="True" w273 {
                    tunnel: [w276 w279] -> w272
                    tunnel: w271 -> [w276 _]
                    tunnel: [TRUE FALSE] -> w270
                    tunnel: w268 -> [_ w277]
                    frame False {
                    }
                    frame True {
                      n82 = case shown="False" w277 {
                        tunnel: [w280 w281] -> w279
                        frame True {
                          w280 = T6[] [enum."Cut After", enum."Generate New Impulse Plot"] items=["Panel Monitoring", "Read Files", "Select Files", "Generate New Impulse Plot", "Impulse Analyser", "Horizontal Align", "Vertical Align", "Vertical Align to Zero", "Delete Trace", "Cut Before", "Cut After", "Filter Data", "Undo Last", "Mean and STD", "Generate Report", "Export Data", "Initialize", "Stop", "Quit"]  # State Stack
                        }
                        frame False {
                          w281 = T6[] [enum."Panel Monitoring"] items=["Panel Monitoring", "Read Files", "Select Files", "Generate New Impulse Plot", "Impulse Analyser", "Horizontal Align", "Vertical Align", "Vertical Align to Zero", "Delete Trace", "Cut Before", "Cut After", "Filter Data", "Undo Last", "Mean and STD", "Generate Report", "Export Data", "Initialize", "Stop", "Quit"]  # State Stack
                        }
                      }
                    }
                  }
                }
                frame 16 {
                  n83 = Unbundle By Name(w288) -> ("Mean and STD"=w287:bool)
                  n84 = Unbundle By Name(w283) -> ("Mean and STD"=w282:bool)
                  n85 = case shown="True" w287 {
                    tunnel: [w290 w293] -> w286
                    tunnel: w285 -> [w290 _]
                    tunnel: [TRUE FALSE] -> w284
                    tunnel: w282 -> [_ w291]
                    frame False {
                    }
                    frame True {
                      n86 = case shown="False" w291 {
                        tunnel: [w294 w295] -> w293
                        frame True {
                          w294 = T6[] [enum."Mean and STD", enum."Panel Monitoring"] items=["Panel Monitoring", "Read Files", "Select Files", "Generate New Impulse Plot", "Impulse Analyser", "Horizontal Align", "Vertical Align", "Vertical Align to Zero", "Delete Trace", "Cut Before", "Cut After", "Filter Data", "Undo Last", "Mean and STD", "Generate Report", "Export Data", "Initialize", "Stop", "Quit"]  # State Stack
                        }
                        frame False {
                          w295 = T6[] [enum."Panel Monitoring"] items=["Panel Monitoring", "Read Files", "Select Files", "Generate New Impulse Plot", "Impulse Analyser", "Horizontal Align", "Vertical Align", "Vertical Align to Zero", "Delete Trace", "Cut Before", "Cut After", "Filter Data", "Undo Last", "Mean and STD", "Generate Report", "Export Data", "Initialize", "Stop", "Quit"]  # State Stack
                        }
                      }
                    }
                  }
                }
                frame 17 {
                  n87 = Unbundle By Name(w303) -> ("Select An  Other Trigger"=w302:bool)
                  n88 = Unbundle By Name(w298) -> ("View Filter Parameters"=w297:bool, "Select An  Other Trigger"=w296:bool)
                  n89 = case shown="True" w302 {
                    tunnel: [w305 w309] -> w301
                    tunnel: w300 -> [w305 _]
                    tunnel: [TRUE FALSE] -> w299
                    tunnel: w297 -> [_ w307]
                    tunnel: w296 -> [_ w306]
                    frame False {
                    }
                    frame True {
                      w309 = T6[] [enum."Panel Monitoring"] items=["Panel Monitoring", "Read Files", "Select Files", "Generate New Impulse Plot", "Impulse Analyser", "Horizontal Align", "Vertical Align", "Vertical Align to Zero", "Delete Trace", "Cut Before", "Cut After", "Filter Data", "Undo Last", "Mean and STD", "Generate Report", "Export Data", "Initialize", "Stop", "Quit"]  # State Stack
                      n90 = Compound Arithmetic op=OR(w307, w306) -> (invert w308:bool)
                      n91 = property on="Trigger Channel" class="Ring (strict)"("Visible"=w306) -> ()  [unwired: 2 in, 2 out]
                      n92 = property on="Group \nAnalyser" class="Bool"("Visible"=w308) -> ()  [unwired: 2 in, 2 out]
                    }
                  }
                }
                frame 18 {
                  n93 = Unbundle By Name(w317) -> ("Export Data"=w316:bool)
                  n94 = Unbundle By Name(w312) -> ("Export Data"=w311:bool)
                  n95 = case shown="True" w316 {
                    tunnel: [w319 w322] -> w315
                    tunnel: w314 -> [w319 _]
                    tunnel: [TRUE FALSE] -> w313
                    tunnel: w311 -> [_ w320]
                    frame False {
                    }
                    frame True {
                      n96 = case shown="True" w320 {
                        tunnel: [w323 w324] -> w322
                        frame True {
                          w323 = T6[] [enum."Export Data", enum."Panel Monitoring"] items=["Panel Monitoring", "Read Files", "Select Files", "Generate New Impulse Plot", "Impulse Analyser", "Horizontal Align", "Vertical Align", "Vertical Align to Zero", "Delete Trace", "Cut Before", "Cut After", "Filter Data", "Undo Last", "Mean and STD", "Generate Report", "Export Data", "Initialize", "Stop", "Quit"]  # State Stack
                        }
                        frame False {
                          w324 = T6[] [enum."Panel Monitoring"] items=["Panel Monitoring", "Read Files", "Select Files", "Generate New Impulse Plot", "Impulse Analyser", "Horizontal Align", "Vertical Align", "Vertical Align to Zero", "Delete Trace", "Cut Before", "Cut After", "Filter Data", "Undo Last", "Mean and STD", "Generate Report", "Export Data", "Initialize", "Stop", "Quit"]  # State Stack
                        }
                      }
                    }
                  }
                }
              }
            }
            n97 = property on="Processing" class="Bool (strict)"("Value"=FALSE) -> ()  [unwired: 2 in, 2 out]
          }
        }
      }
      frame "Select Files" {
        w332 = "*.lvd" ("pattern")
        (unwired) T11."existing dir" ("select mode (2)")
        w335 = T6[] [enum."Panel Monitoring"] items=["Panel Monitoring", "Read Files", "Select Files", "Generate New Impulse Plot", "Impulse Analyser", "Horizontal Align", "Vertical Align", "Vertical Align to Zero", "Delete Trace", "Cut Before", "Cut After", "Filter Data", "Undo Last", "Mean and STD", "Generate Report", "Export Data", "Initialize", "Stop", "Quit"]
        n98 = File Dialog(6:w332, 7:"Select A Directory" ("prompt")) -> (0:w325:errorcluster, 3:w334:path)  [unwired: 5 in, 2 out]
        n99 = Unbundle(w325) -> ()  [unwired: 3 out]
        n100 = List Folder(path=w334, pattern=w332) -> (path out=w330:path, filenames=w331:string[])  [unwired: 2 in, 2 out]
        n101 = Path To String(path=w330) -> (string=w329:string)
        n102 = for {
          tunnel: w331 -> [w341] mode=indexing
          tunnel: w329 -> [w340]
          tunnel: [w338] -> w327 mode=indexing
          n103 = Concatenate Strings(w340, "\\" ("Substring"), w341) -> (w338:string)
        }
        n104 = local write "Selected Files Text"(w327) -> ()
        n105 = property on="Listbox" class="LstBox (strict)"("Item Names"=w327) -> ()  [unwired: 2 in, 2 out]
        n106 = Bundle By Name(cluster=w328, "Selected Files Text"=w327) -> (w326:T9)
      }
      frame "Read Files" {
        w357 = T6[] [enum."Panel Monitoring"] items=["Panel Monitoring", "Read Files", "Select Files", "Generate New Impulse Plot", "Impulse Analyser", "Horizontal Align", "Vertical Align", "Vertical Align to Zero", "Delete Trace", "Cut Before", "Cut After", "Filter Data", "Undo Last", "Mean and STD", "Generate Report", "Export Data", "Initialize", "Stop", "Quit"]
        n107 = Unbundle By Name(w356) -> ("Selected Files Text"=w354:string[])
        n108 = local read "Data Input"() -> (w353:T2)
        n109 = Index Array(array=w353, index=0 ("Index")) -> (element=w351:T12)
        n110 = for {
          tunnel: "Listbox" -> [w364] mode=indexing
          tunnel: w354 -> [w365]
          tunnel: w351 -> [w361]
          tunnel: [w360] -> w347 mode=indexing
          w367 = 4 ("count")
          n111 = Index Array(array=w365, index=w364) -> (element=w363:string)
          n112 = String To Path(string=w363) -> (path=w362:path)
          n113 = call <vilib>:"Open_Create_Replace File.vi"("file path"=w362) -> ("refnum"=w370:refnum<file>)  [unwired: 7 in, 3 out]
          n114 = call <vilib>:"Read File+ (string).vi"("count"=w367, "refnum"=w370) -> ("string"=w368:string, "dup refnum"=w369:refnum<file>)  [unwired: 5 in, 3 out]
          n115 = Unflatten From String(type=w367, binary string=w368) -> (value=w366:i32)  [unwired: 3 in, 2 out]
          n116 = call <vilib>:"Read File+ (string).vi"("count"=w366, "refnum"=w369) -> ("string"=w371:string)  [unwired: 5 in, 4 out]
          n117 = Unflatten From String(type=w361, binary string=w371) -> (value=w360:T12)  [unwired: 3 in, 2 out]
        }
        n118 = local write "Data Input"(w347) -> ()
        n119 = Index Array(array=w347, index=0 ("Index")) -> (element=w348:T12)
        n120 = Unbundle By Name(w348) -> ("Channel List"=w346:string[])
        n121 = Array Size(array=w346) -> (size(s)=w344:i32)
        n122 = Array Size(array=w347) -> (size(s)=w345:i32)
        n123 = Initialize Array(T7 {"Start"=0, "End"=100000, "Offset"=0, "Deleted"=FALSE} ("Cluster"), w344, w345) -> (w343:T13)
        n124 = Bundle By Name(cluster=w356, "Channels / Subject"=w343, "Data Input"=w347) -> (w350:T9)
        n125 = property on="List 1" class="Ring (strict)"("Strings []"=w346) -> ()  [unwired: 2 in, 2 out]
        n126 = property on="List 2" class="Ring (strict)"("Strings []"=w346) -> ()  [unwired: 2 in, 2 out]
        n127 = property on="Trigger Channel" class="Ring (strict)"("Strings []"=w346) -> ()  [unwired: 2 in, 2 out]
        n128 = property on="Aligning Channel" class="Ring (strict)"("Strings []"=w346) -> ()  [unwired: 2 in, 2 out]
        n129 = local write "Channels / Subject"(w343) -> ()
      }
      frame "Filter Data" {
        n130 = Unbundle By Name("Filter characteristics") -> ("Lower pass freq"=w377:dbl, "Higher pass freq"=w378:dbl, "Filter type"=w380:T14, "Order"=w379:i32)
        n131 = Unbundle By Name(w373) -> ("Data Input"=w376:T2)
        n132 = for {
          tunnel: w380 -> [w392]
          tunnel: w379 -> [w391]
          tunnel: w378 -> [w390]
          tunnel: w377 -> [w389]
          tunnel: w376 -> [w386] mode=indexing
          tunnel: [w384] -> w374 mode=indexing
          n133 = Unbundle By Name(w386) -> ("Data Channels"=w388:dbl[][], "Sample Rate"=w387:i32)
          n134 = call "FIR filter neu.vi"("order"=w391, "filter type"=w392, "higher pass freq"=w390, "lower pass freq"=w389, "sampling freq: fs"=w387, "3D Unfiltered Data"=w388) -> ("Output Array"=w385:dbl[][])  [unwired: 3 in]
          n135 = Bundle By Name(cluster=w386, "Data Channels"=w385) -> (w384:T12)
        }
        n136 = local write "Data Input"(w374) -> ()
        n137 = Bundle By Name(cluster=w373, "Data Input"=w374) -> (w372:T9)
      }
      frame "Generate New Impulse Plot" {
        w403 = T6[] [enum."Panel Monitoring"] items=["Panel Monitoring", "Read Files", "Select Files", "Generate New Impulse Plot", "Impulse Analyser", "Horizontal Align", "Vertical Align", "Vertical Align to Zero", "Delete Trace", "Cut Before", "Cut After", "Filter Data", "Undo Last", "Mean and STD", "Generate Report", "Export Data", "Initialize", "Stop", "Quit"]
        n138 = Unbundle By Name(w398) -> ("Data Input"=w395:T2, "Channels / Subject"=w393:T1)
        n139 = Index Array(array=w395, index=0 ("Index")) -> (element=w399:T12)
        n140 = Unbundle By Name(w399) -> ("Sample Rate"=w402:i32)
        n141 = Array Size(array=w395) -> (size(s)=w396:i32)
        n142 = To Double Precision Float(number=w402) -> (double precision float=w401:dbl)
        n143 = stacked-sequence {
          tunnel: w396 -> [_ _ w435]
          tunnel: "Plot Selection 2" -> [_ w430 w437]
          tunnel: w401 -> [_ w433 _]
          tunnel: w393 -> [_ w424 w434]
          tunnel: w395 -> [_ w425 _]
          tunnel: "Plot Selection" -> [_ w423 w436]
          frame #0 {
            n144 = case shown="False" "Fixed Time" {
              tunnel: [u8 0 ("Y Scale.Scale Fit") u8 2 ("Y Scale.Scale Fit")] -> w409
              frame True {
              }
              frame False {
              }
            }
            n145 = case shown="False" "Fixed Amplitude" {
              tunnel: [u8 0 ("Y Scale.Scale Fit") u8 2 ("Y Scale.Scale Fit")] -> w412
              frame True {
              }
              frame False {
              }
            }
            n146 = case shown="False" "Fixed Amplitude" {
              tunnel: [u8 0 ("Y Scale.Scale Fit") u8 2 ("Y Scale.Scale Fit")] -> w411
              frame True {
              }
              frame False {
              }
            }
            n147 = case shown="False" "Fixed Time" {
              tunnel: [u8 0 ("Y Scale.Scale Fit") u8 2 ("Y Scale.Scale Fit")] -> w407
              frame True {
              }
              frame False {
              }
            }
            n148 = property on="Impulse Trace" class="WFGraph (strict)"("X Scale.Scale Fit"=w409) -> ()  [unwired: 2 in, 2 out]
            n149 = property on="Impulse Trace" class="WFGraph (strict)"("Y Scale.Scale Fit"=w412) -> ()  [unwired: 2 in, 2 out]
            n150 = property on="Impulse Trace" class="WFGraph (strict)"("Y Scale.Scale Fit"=w411) -> ()  [unwired: 2 in, 2 out]
            n151 = property on="Impulse Trace" class="WFGraph (strict)"("X Scale.Scale Fit"=w407) -> ()  [unwired: 2 in, 2 out]
          }
          frame #1 {
            w429 = 0.0
            n152 = call "Group Traces.vi"("Plot Selection 2"=w430, "Channels / Subject"=w424, "Data Input"=w425) -> ("Output"=w426:dbl[][])  [unwired: 5 in, 2 out]
            n153 = call "Group Traces.vi"("Plot Selection 2"=w423, "Channels / Subject"=w424, "Data Input"=w425) -> ("Output"=w422:dbl[][])  [unwired: 5 in, 2 out]
            n154 = Divide(x=1000.0 ("y"), y=w433) -> (x/y=w428:dbl)
            n155 = Bundle(w429, w428, "Output"=w426) -> (→"Impulse Trace":cluster{dbl, dbl, "Output":dbl[][]})  [unwired: 1 in]
            n156 = Bundle(w429, w428, "Output"=w422) -> (→"Impulse Trace":cluster{dbl, dbl, "Output":dbl[][]})  [unwired: 1 in]
          }
          frame #2 {
            n157 = for {
              tunnel: w436 -> [w445] mode=indexing
              tunnel: w435 -> [w443]
              tunnel: w434 -> [w438]
              i -> [w444]
              n158 = Unbundle By Name(w445) -> ("Color Box"=w441:u32, "Boolean"=w440:bool, "List 1"=w439:u16)
              n159 = Multiply(x=w443, y=w444) -> (x*y=w442:i32)
              n160 = for {
                N: w443 -> [_]
                tunnel: w442 -> [w456]
                tunnel: w441 -> [w448]
                tunnel: w440 -> [w450]
                tunnel: w439 -> [w455]
                tunnel: w438 -> [w452]
                i -> [w454]
                n161 = Add(x=w454, y=w456) -> (x+y=w449:i32)
                n162 = Index Array(array=w452, index (row)=w455, index (col)=w454) -> (element=w453:T15)
                n163 = Unbundle By Name(w453) -> ("Deleted"=w451:bool)
                n164 = case shown="False" w451 {
                  tunnel: w450 -> [w457 _]
                  tunnel: [w457 FALSE ("Boolean")] -> w447
                  frame False {
                  }
                  frame True {
                  }
                }
                n165 = property on="Impulse Trace" class="WFGraph (strict)"("Active Plot"=w449, "Plot.Plot Color"=w448, "Plot.Visible"=w447, "Plot.Line Width"=u8 0) -> ()  [unwired: 2 in, 2 out]
              }
            }
            n166 = for {
              tunnel: w437 -> [w466] mode=indexing
              tunnel: w435 -> [w464]
              tunnel: w434 -> [w460]
              i -> [w465]
              n167 = Unbundle By Name(w466) -> ("Color Box"=w462:u32, "Boolean"=w461:bool, "List 2"=w459:u16)
              n168 = Multiply(x=w464, y=w465) -> (x*y=w463:i32)
              n169 = for {
                N: w464 -> [_]
                tunnel: w463 -> [w477]
                tunnel: w462 -> [w473]
                tunnel: w461 -> [w468]
                tunnel: w460 -> [w474]
                tunnel: w459 -> [w472]
                i -> [w471]
                n170 = Add(x=w471, y=w477) -> (x+y=w476:i32)
                n171 = Index Array(array=w474, index (row)=w472, index (col)=w471) -> (element=w470:T15)
                n172 = Unbundle By Name(w470) -> ("Deleted"=w469:bool)
                n173 = case shown="False" w469 {
                  tunnel: w468 -> [w478 _]
                  tunnel: [w478 FALSE ("Boolean")] -> w467
                  frame False {
                  }
                  frame True {
                  }
                }
                n174 = property on="Impulse Trace" class="WFGraph (strict)"("Active Plot"=w476, "Plot.Plot Color"=w473, "Plot.Visible"=w467, "Plot.Line Width"=u8 0) -> ()  [unwired: 2 in, 2 out]
              }
            }
          }
        }
      }
      frame "Horizontal Align" {
        n175 = Unbundle By Name(w489) -> ("Data Input"=w487:T2, "Channels / Subject"=w484:T1)
        n176 = case shown="0, Default" "Active Plot" {
          tunnel: [w494 w496] -> w481
          tunnel: [w493 w495] -> w480
          frame 0, Default {
            n177 = property on="Impulse Trace" class="WFGraph (strict)"() -> ("Cursor.Cursor Position:Cursor X"=w494:dbl, "Cursor.Cursor Position:Cursor Y"=w493:dbl)  [unwired: 2 in, 2 out]
          }
          frame 1 {
            n178 = property on="Impulse Trace" class="WFGraph (strict)"() -> ("Cursor.Cursor Position:Cursor X"=w496:dbl, "Cursor.Cursor Position:Cursor Y"=w495:dbl)  [unwired: 2 in, 2 out]
          }
        }
        n179 = call "Align Traces.vi"("Data Input"=w487, "Alignment"=enum16{"Vertically", "Horizontally"}."Horizontally", "Aligning Channel"="Aligning Channel", "Y Level"=w480, "X Level"=w481, "Channels / Subject (in)"=w484) -> ("Channels / Subject (out)"=w483:T1)  [unwired: 13 in]
        n180 = local write "Old Channels / Subject"(w484) -> ()
        n181 = local write "Channels / Subject"(w483) -> ()
        n182 = Bundle By Name(cluster=w489, "Channels / Subject"=w483, "Old Channels / Subject"=w484) -> (w488:T9)
      }
      frame "Vertical Align" {
        n183 = Unbundle By Name(w504) -> ("Data Input"=w506:T2, "Channels / Subject"=w500:T1)
        n184 = local read "Active Plot"() -> (w497:u16)
        n185 = case shown="0, Default" w497 {
          tunnel: [w511 w513] -> w499
          tunnel: [w510 w512] -> w498
          frame 0, Default {
            n186 = property on="Impulse Trace" class="WFGraph (strict)"() -> ("Cursor.Cursor Position:Cursor X"=w511:dbl, "Cursor.Cursor Position:Cursor Y"=w510:dbl)  [unwired: 2 in, 2 out]
          }
          frame 1 {
            n187 = property on="Impulse Trace" class="WFGraph (strict)"() -> ("Cursor.Cursor Position:Cursor X"=w513:dbl, "Cursor.Cursor Position:Cursor Y"=w512:dbl)  [unwired: 2 in, 2 out]
          }
        }
        n188 = local read "Aligning Channel"() -> (w502:u16)
        n189 = call "Align Traces.vi"("Data Input"=w506, "Alignment"=enum16{"Vertically", "Horizontally"}."Vertically", "Aligning Channel"=w502, "Y Level"=w498, "X Level"=w499, "Channels / Subject (in)"=w500) -> ("Channels / Subject (out)"=w501:T1)  [unwired: 13 in]
        n190 = local write "Old Channels / Subject"(w500) -> ()
        n191 = local write "Channels / Subject"(w501) -> ()
        n192 = Bundle By Name(cluster=w504, "Channels / Subject"=w501, "Old Channels / Subject"=w500) -> (w503:T9)
      }
      frame "Vertical Align to Zero" {
        n193 = Unbundle By Name(w520) -> ("Data Input"=w521:T2, "Channels / Subject"=w517:T1)
        n194 = local read "Active Plot"() -> (w515:u16)
        n195 = case shown="1" w515 {
          tunnel: [w526 w528] -> w514
          tunnel: [w525 w527] -> _
          frame 0, Default {
            n196 = property on="Impulse Trace" class="WFGraph (strict)"() -> ("Cursor.Cursor Position:Cursor X"=w526:dbl, "Cursor.Cursor Position:Cursor Y"=w525:dbl)  [unwired: 2 in, 2 out]
          }
          frame 1 {
            n197 = property on="Impulse Trace" class="WFGraph (strict)"() -> ("Cursor.Cursor Position:Cursor X"=w528:dbl, "Cursor.Cursor Position:Cursor Y"=w527:dbl)  [unwired: 2 in, 2 out]
          }
        }
        n198 = call "Align Traces to Zero.vi"("Data Input"=w521, "Y Level"=0.0 ("X Level"), "X Level"=w514, "Channels / Subject (in)"=w517) -> ("Channels / Subject (out)"=w518:T1)  [unwired: 15 in]
        n199 = local write "Old Channels / Subject"(w517) -> ()
        n200 = local write "Channels / Subject"(w518) -> ()
        n201 = Bundle By Name(cluster=w520, "Channels / Subject"=w518, "Old Channels / Subject"=w517) -> (w519:T9)
      }
      frame "Cut Before" {
        n202 = local read "Active Plot"() -> (w530:u16)
        n203 = case shown="0, Default" w530 {
          tunnel: [w543 w545] -> w529
          tunnel: [w542 w544] -> _
          frame 0, Default {
            n204 = property on="Impulse Trace" class="WFGraph (strict)"() -> ("Cursor.Cursor Position:Cursor X"=w543:dbl, "Cursor.Cursor Position:Cursor Y"=w542:dbl)  [unwired: 2 in, 2 out]
          }
          frame 1 {
            n205 = property on="Impulse Trace" class="WFGraph (strict)"() -> ("Cursor.Cursor Position:Cursor X"=w545:dbl, "Cursor.Cursor Position:Cursor Y"=w544:dbl)  [unwired: 2 in, 2 out]
          }
        }
        n206 = Unbundle By Name(w537) -> ("Channels / Subject"=w532:T1, "Data Input"=w536:T2)
        n207 = Index Array(array=w536, index=0 ("Index")) -> (element=w534:T12)
        n208 = Unbundle By Name(w534) -> ("Sample Rate"=w533:i32)
        n209 = for {
          tunnel: w532 -> [w549] mode=indexing
          tunnel: [w548] -> w531 mode=indexing
          tunnel: w529 -> [w547]
          tunnel: w533 -> [w546]
          n210 = for {
            tunnel: w549 -> [w555] mode=indexing
            tunnel: [w554] -> w548 mode=indexing
            tunnel: w547 -> [w551]
            tunnel: w546 -> [w550]
            n211 = Divide(x=w550, y=1000) -> (x/y=w558:dbl)
            n212 = Multiply(x=w558, y=w551) -> (x*y=w556:dbl)
            n213 = To Long Integer(number=w556) -> (32bit integer=w557:i32)
            n214 = Unbundle By Name(w555) -> ("Start"=w553:i32)
            n215 = Add(x=w553, y=w557) -> (x+y=w552:i32)
            n216 = Bundle By Name(cluster=w555, "Start"=w552) -> (w554:T15)
          }
        }
        n217 = local write "Old Channels / Subject"(w532) -> ()
        n218 = local write "Channels / Subject"(w531) -> ()
        n219 = Bundle By Name(cluster=w537, "Old Channels / Subject"=w532, "Channels / Subject"=w531) -> (w539:T9)
      }
      frame "Cut After" {
        n220 = local read "Active Plot"() -> (w561:u16)
        n221 = case shown="0, Default" w561 {
          tunnel: [w574 w576] -> w560
          tunnel: [w573 w575] -> _
          frame 0, Default {
            n222 = property on="Impulse Trace" class="WFGraph (strict)"() -> ("Cursor.Cursor Position:Cursor X"=w574:dbl, "Cursor.Cursor Position:Cursor Y"=w573:dbl)  [unwired: 2 in, 2 out]
          }
          frame 1 {
            n223 = property on="Impulse Trace" class="WFGraph (strict)"() -> ("Cursor.Cursor Position:Cursor X"=w576:dbl, "Cursor.Cursor Position:Cursor Y"=w575:dbl)  [unwired: 2 in, 2 out]
          }
        }
        n224 = Unbundle By Name(w563) -> ("Channels / Subject"=w565:T1, "Data Input"=w569:T2)
        n225 = Index Array(array=w569, index=0 ("Index")) -> (element=w567:T12)
        n226 = Unbundle By Name(w567) -> ("Sample Rate"=w566:i32)
        n227 = for {
          tunnel: w565 -> [w580] mode=indexing
          tunnel: [w579] -> w564 mode=indexing
          tunnel: w560 -> [w578]
          tunnel: w566 -> [w577]
          n228 = for {
            tunnel: w580 -> [w586] mode=indexing
            tunnel: [w585] -> w579 mode=indexing
            tunnel: w578 -> [w582]
            tunnel: w577 -> [w581]
            n229 = Divide(x=w581, y=1000) -> (x/y=w589:dbl)
            n230 = Multiply(x=w589, y=w582) -> (x*y=w587:dbl)
            n231 = To Long Integer(number=w587) -> (32bit integer=w588:i32)
            n232 = Unbundle By Name(w586) -> ("Start"=w584:i32)
            n233 = Add(x=w584, y=w588) -> (x+y=w583:i32)
            n234 = Bundle By Name(cluster=w586, "End"=w583) -> (w585:T15)
          }
        }
        n235 = local write "Old Channels / Subject"(w565) -> ()
        n236 = local write "Channels / Subject"(w564) -> ()
        n237 = Bundle By Name(cluster=w563, "Old Channels / Subject"=w565, "Channels / Subject"=w564) -> (w562:T9)
      }
      frame "Undo Last" {
        n238 = Unbundle By Name(w594) -> ("Old Channels / Subject"=w591:T1)
        n239 = local write "Channels / Subject"(w591) -> ()
        n240 = Bundle By Name(cluster=w594, "Channels / Subject"=w591) -> (w593:T9)
      }
      frame "Delete Trace" {
        n241 = Unbundle By Name(w609) -> ("Channels / Subject"=w607:T1)  [unwired: 1 out]
        n242 = Array Size(array=w607) -> (size(s)=w602:i32[])
        n243 = local read "Active Plot"() -> (w597:u16)
        n244 = Index Array(array=w602, index=1 ("Index")) -> (element=w600:i32)
        n245 = case shown="0, Default" w597 {
          tunnel: [w616 w625] -> w604
          tunnel: w600 -> [w614 w623]
          tunnel: [w613 w622] -> w599
          frame 0, Default {
            n246 = property on="Impulse Trace" class="WFGraph (strict)"() -> ("Cursor.Cursor Plot"=w619:i32)  [unwired: 2 in, 2 out]
            n247 = Quotient & Remainder(x=w619, y=w614) -> (x-y*floor(x/y)=w613:i32, floor(x/y)=w615:i32)
            n248 = local read "Plot Selection 2"() -> (w618:T3)
            n249 = Index Array(array=w618, index=w615) -> (element=w617:T16)
            n250 = Unbundle By Name(w617) -> ("List 2"=w616:u16)
          }
          frame 1 {
            n251 = property on="Impulse Trace" class="WFGraph (strict)"() -> ("Cursor.Cursor Plot"=w621:i32)  [unwired: 2 in, 2 out]
            n252 = Quotient & Remainder(x=w621, y=w623) -> (x-y*floor(x/y)=w622:i32, floor(x/y)=w624:i32)
            n253 = local read "Plot Selection"() -> (w620:T5)
            n254 = Index Array(array=w620, index=w624) -> (element=w626:T17)
            n255 = Unbundle By Name(w626) -> ("List 1"=w625:u16)
          }
        }
        n256 = Index Array(array=w607, index (row)=w604, index (col)=w599) -> (element=w606:T15)
        n257 = Bundle By Name(cluster=w606, "Deleted"=TRUE) -> (w603:T15)
        n258 = Replace Array Subset(array=w607, new element=w603, index (row)=w604, index (col)=w599) -> (w598:T1)
        n259 = local write "Old Channels / Subject"(w607) -> ()
        n260 = local write "Channels / Subject"(w598) -> ()
        n261 = Bundle By Name(cluster=w609, "Channels / Subject"=w598, "Old Channels / Subject"=w607) -> (w608:T9)
      }
      frame "Mean and STD" {
        w636 = T6[] [enum."Panel Monitoring"] items=["Panel Monitoring", "Read Files", "Select Files", "Generate New Impulse Plot", "Impulse Analyser", "Horizontal Align", "Vertical Align", "Vertical Align to Zero", "Delete Trace", "Cut Before", "Cut After", "Filter Data", "Undo Last", "Mean and STD", "Generate Report", "Export Data", "Initialize", "Stop", "Quit"]
        n262 = Unbundle By Name(w631) -> ("Data Input"=w627:T2, "Channels / Subject"=w630:T1)
        n263 = local read "Plot Selection 2"() -> (w629:T3)
        n264 = Index Array(array=w627, index=0 ("Index")) -> (element=w632:T12)
        n265 = Unbundle By Name(w632) -> ("Sample Rate"=w635:i32)
        n266 = local read "Plot Selection"() -> (w628:T5)
        n267 = To Double Precision Float(number=w635) -> (double precision float=w634:dbl)
        n268 = stacked-sequence {
          tunnel: w629 -> [_ w657 w661]
          tunnel: w634 -> [_ w659 _]
          tunnel: w630 -> [_ w652 _]
          tunnel: w627 -> [_ w653 _]
          tunnel: w628 -> [_ w651 w660]
          frame #0 {
            n269 = local read "Fixed Amplitude"() -> (w640:bool)
            n270 = local read "Fixed Amplitude"() -> (w639:bool)
            n271 = case shown="False" w640 {
              tunnel: [u8 0 ("Y Scale.Scale Fit") u8 2 ("Y Scale.Scale Fit")] -> w642
              frame True {
              }
              frame False {
              }
            }
            n272 = case shown="False" w639 {
              tunnel: [u8 0 ("Y Scale.Scale Fit") u8 2 ("Y Scale.Scale Fit")] -> w641
              frame True {
              }
              frame False {
              }
            }
            n273 = property on="Impulse Trace" class="WFGraph (strict)"("Y Scale.Scale Fit"=w642) -> ()  [unwired: 2 in, 2 out]
            n274 = property on="Impulse Trace" class="WFGraph (strict)"("Y Scale.Scale Fit"=w641) -> ()  [unwired: 2 in, 2 out]
          }
          frame #1 {
            w647 = TRUE ("Mean")
            w656 = 0.0
            n275 = call "Group Traces.vi"("Mean"=w647, "Plot Selection 2"=w657, "Channels / Subject"=w652, "Data Input"=w653) -> ("Output"=w654:dbl[][])  [unwired: 4 in, 2 out]
            n276 = call "Group Traces.vi"("Mean"=w647, "Plot Selection 2"=w651, "Channels / Subject"=w652, "Data Input"=w653) -> ("Output"=w650:dbl[][])  [unwired: 4 in, 2 out]
            n277 = Divide(x=1000.0 ("y"), y=w659) -> (x/y=w655:dbl)
            n278 = Bundle(w656, w655, "Output"=w654) -> (w649:cluster{dbl, dbl, "Output":dbl[][]})  [unwired: 1 in]
            n279 = Bundle(w656, w655, "Output"=w650) -> (w648:cluster{dbl, dbl, "Output":dbl[][]})  [unwired: 1 in]
            n280 = local write "Impulse Trace"(w648) -> ()
            n281 = local write "Impulse Trace"(w649) -> ()
          }
          frame #2 {
            n282 = for {
              tunnel: w660 -> [w667] mode=indexing
              i -> [w666]
              w662 = 3  # M-STD, M, M+STD
              n283 = Unbundle By Name(w667) -> ("Color Box"=w664:u32, "Boolean"=w663:bool)
              n284 = Multiply(x=w662, y=w666) -> (x*y=w665:i32)
              n285 = for {
                N: w662 -> [_]
                tunnel: w665 -> [w675]
                tunnel: w664 -> [w670]
                tunnel: w663 -> [w669]
                i -> [w673]
                n286 = Add(x=w673, y=w675) -> (x+y=w671:i32)
                n287 = Equal?(x=w673, y=1) -> (x = y?=w674:bool)
                n288 = case shown="True" w674 {
                  tunnel: [u8 0 ("Plot.Line Width") u8 5 ("Plot.Line Width")] -> w668
                  frame False {
                  }
                  frame True {
                  }
                }
                n289 = property on="Impulse Trace" class="WFGraph (strict)"("Active Plot"=w671, "Plot.Plot Color"=w670, "Plot.Visible"=w669, "Plot.Line Width"=w668) -> ()  [unwired: 2 in, 2 out]
              }
            }
            n290 = for {
              tunnel: w661 -> [w683] mode=indexing
              i -> [w682]
              w678 = 3  # M-STD, M, M+STD
              n291 = Unbundle By Name(w683) -> ("Color Box"=w680:u32, "Boolean"=w679:bool)
              n292 = Multiply(x=w678, y=w682) -> (x*y=w681:i32)
              n293 = for {
                N: w678 -> [_]
                tunnel: w681 -> [w691]
                tunnel: w680 -> [w690]
                tunnel: w679 -> [w689]
                i -> [w687]
                n294 = Add(x=w687, y=w691) -> (x+y=w685:i32)
                n295 = Equal?(x=w687, y=1) -> (x = y?=w688:bool)
                n296 = case shown="True" w688 {
                  tunnel: [u8 0 ("Plot.Line Width") u8 5 ("Plot.Line Width")] -> w684
                  frame False {
                  }
                  frame True {
                  }
                }
                n297 = property on="Impulse Trace" class="WFGraph (strict)"("Active Plot"=w685, "Plot.Plot Color"=w690, "Plot.Visible"=w689, "Plot.Line Width"=w684) -> ()  [unwired: 2 in, 2 out]
              }
            }
          }
        }
      }
      frame "Impulse Analyser" {
      }
      frame "Export Data" {
        (unwired) T11."new or existing file" ("select mode (2)")
        w717 = "\r"
        w733 = "\r"
        w742 = T6[] [enum."Panel Monitoring"] items=["Panel Monitoring", "Read Files", "Select Files", "Generate New Impulse Plot", "Impulse Analyser", "Horizontal Align", "Vertical Align", "Vertical Align to Zero", "Delete Trace", "Cut Before", "Cut After", "Filter Data", "Undo Last", "Mean and STD", "Generate Report", "Export Data", "Initialize", "Stop", "Quit"]
        n298 = Unbundle By Name(w741) -> ("Channels / Subject"=w702:T1, "Data Input"=w703:T2)
        n299 = local read "Plot Selection 2"() -> (w740:T3)
        n300 = Index Array(array=w703, index=0 ("Index")) -> (element=w706:T12)
        n301 = Index Array(array=w740, index=0 ("Index")) -> (element=w738:T16)
        n302 = Unbundle By Name(w706) -> ("Sample Rate"=w705:i32, "Channel List"=w704:string[])
        n303 = Array Size(array=w704) -> (size(s)=w729:i32)
        n304 = for {
          tunnel: w738 -> [w751]
          tunnel: [w749] -> w701 mode=indexing
          shift-right: [w747] -> w718
          shift-left: "" -> [w748]
          tunnel: w704 -> [w746] mode=indexing
          i -> [w750]
          n305 = Bundle By Name(cluster=w751, "List 2"=w750) -> (w749:T16)
          n306 = Concatenate Strings(w748, w746, "\t") -> (w747:string)
        }
        n307 = Format Into String(format string="%d" ("Format String"), w729) -> (resulting string=w727:string)  [unwired: 2 in, 1 out]
        n308 = To Double Precision Float(number=w705) -> (double precision float=w737:dbl)
        n309 = call "Group Traces.vi"("Mean"=TRUE, "Plot Selection 2"=w701, "Channels / Subject"=w702, "Data Input"=w703) -> ("Mean"=w699:dbl[][])  [unwired: 4 in, 2 out]
        n310 = Format Into String(format string="%d" ("Format String"), w737) -> (resulting string=w735:string)  [unwired: 2 in, 1 out]
        n311 = Concatenate Strings("Number of Channels " ("Substring"), w727, w717, "Channel  Names " ("Substring"), w717, w718) -> (w734:string)
        n312 = Concatenate Strings("Sample Rate ", w735, w733, w734, w733) -> (w720:string)
        n313 = File Dialog(7:"Please Enter Name Of File (NO Postfix):" ("prompt")) -> (0:w698:errorcluster, 3:w710:path)  [unwired: 6 in, 2 out]
        n314 = Transpose 2D Array "Means"(2D array=w699) -> (transposed array=w726:dbl[][])
        n315 = Unbundle(w698) -> ()  [unwired: 3 out]
        n316 = Path To String(path=w710) -> (string=w709:string)
        n317 = Concatenate Strings(w709, ".txt" ("Substring")) -> (w712:string)
        n318 = Array To Spreadsheet String(delimiter (Tab)="\t", array=w726, 3:"%.5f" ("format string")) -> (spreadsheet string=w723:string)
        n319 = String To Path(string=w712) -> (path=w711:path)
        n320 = call <vilib>:"Open_Create_Replace File.vi"("function (open:0)"=T8."create or replace", "file path"=w711) -> ("error out"=w716:errorcluster, "refnum"=w715:refnum<file>)  [unwired: 6 in, 2 out]
        n321 = call <vilib>:"Write File+ (string).vi"("string"=w720, "error in (no error)"=w716, "refnum"=w715) -> ("dup refnum"=w722:refnum<file>)  [unwired: 4 in, 2 out]
        n322 = call <vilib>:"Write File+ (string).vi"("string"=w723, "refnum"=w722) -> ("dup refnum"=w721:refnum<file>)  [unwired: 5 in, 2 out]
        n323 = call <vilib>:"Close File+.vi"("refnum"=w721) -> ()  [unwired: 4 in, 3 out]
      }
      frame "Generate Report" {
        w753 = T6[] [enum."Panel Monitoring"] items=["Panel Monitoring", "Read Files", "Select Files", "Generate New Impulse Plot", "Impulse Analyser", "Horizontal Align", "Vertical Align", "Vertical Align to Zero", "Delete Trace", "Cut Before", "Cut After", "Filter Data", "Undo Last", "Mean and STD", "Generate Report", "Export Data", "Initialize", "Stop", "Quit"]
      }
    }
  }
